vi "VolumeScan.vi"() -> ()   [LabVIEW 2018]
uses:
  <vilib>/Utility/miscctls.llb/LVRowAndColumnTypeDef.ctl
  <vilib>/vision/NI_Vision_Development_Module.lvlib
panel:
  in  "Graph parameters":T1={"Graph type"=1, "Scale"=1.0, "Offset"=0.0, "Automatic"=""} {"Graph type" items=["Mean(Y)", "Mean(X)"]}
  out "Image":T2(plugin-control)
  out "XY Graph":cluster{"X":dbl, "Y":dbl}[](graph)
  out "Status":string
  in  "Capture":bool
  in  "Tab Control":T3(tab)
  in  "Graph settings":bool
  in  "Close camera":bool
  in  "Display":u16(ring) items=["Image", "Graph", "Volume"]
  in  "Frames per position":u32=1 min=1 step=1
  in  "Camera settings":bool
  out "Status":bool
  out "Temperature":dbl
  in  "Camera identity":u16(ring)=1 items=["Andor", "Dummy", "PCO Edge", "PointGrey Grasshopper Temp", "PointGrey Grasshopper"]
  in  "Exposure (s)":dbl=0.1
  in  "16-bit mapping":u16(ring) items=["Full range", "Full dynamic", "90% dynamic", "Fixed"]
  in  "16 bit low":i32
  in  "16 bit high":i32=65535
  in  "Camera settings table":i32(listbox)=-1
  in  "Open camera":bool
  in  "Wizards":i32(ring) items=["Circle", "Function"]
  in  "Volume Wizard":bool
  in  "Imaging Locations":dbl[][](array[numeric])
  in  "Device positions":dbl[](array[numeric]) format="%_5g"
  in  "Save":T4(ring)
  in  "Path":path=path "G:/"
  in  "File Prefix":string="Prefix"
  in  "Configure device":bool
  in  "Close device":bool
  in  "Device Settings":i32(listbox)=-1
  in  "Open device":bool
  in  "Shut Down":bool
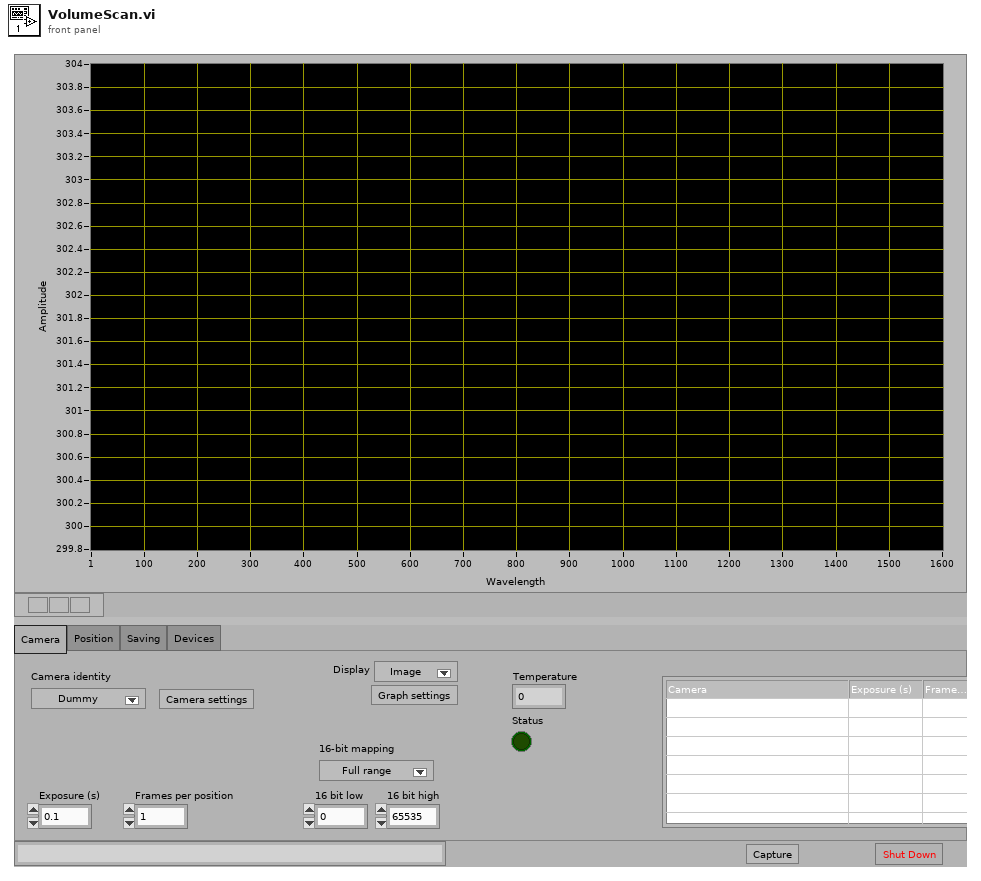
[diagram p1: front panel]
types:
  T1 = cluster{"Graph type":u16, "Scale":dbl, "Offset":dbl, "Automatic":string}
  T2 = typedef "IMAQ Image.ctl" = refnum<image>
  T3 = enum32{"Camera", "Position", "Saving", "Devices"}
  T4 = enum16{"Don't save", "Save U16", "Save PNG", "Save TIFF"}
  T5 = typedef "LVRowAndColumnTypeDef.ctl" = cluster{"Row":i32, "Column":i32}
  T6 = enum16{"Initialize", "Shut down", "Set capture mode", "Set exposure", "Trigger and read", "Get status", "Other settings"}
  T7 = typedef "Image Type" = u32
  T8 = enum16{"Initialize", "Shut down", "Set position", "Get position", "Get status", "Other settings"}
  T9 = cluster{"System OK?":bool, "Current exposure":dbl, "Temperature":dbl, "ROI":cluster{"X":u32, "X2":u32, "Y":u32, "Y2":u32}, "Binning":cluster{"X":u32, "Y":u32}}
  T10 = cluster{"System OK?":bool, "Temperature":dbl, "Limit switch high":bool[], "Limit switch low":bool[]}
  T11 = typedef "LVPoint32TypeDef.ctl" = cluster{"Horizontal":i32, "Vertical":i32}
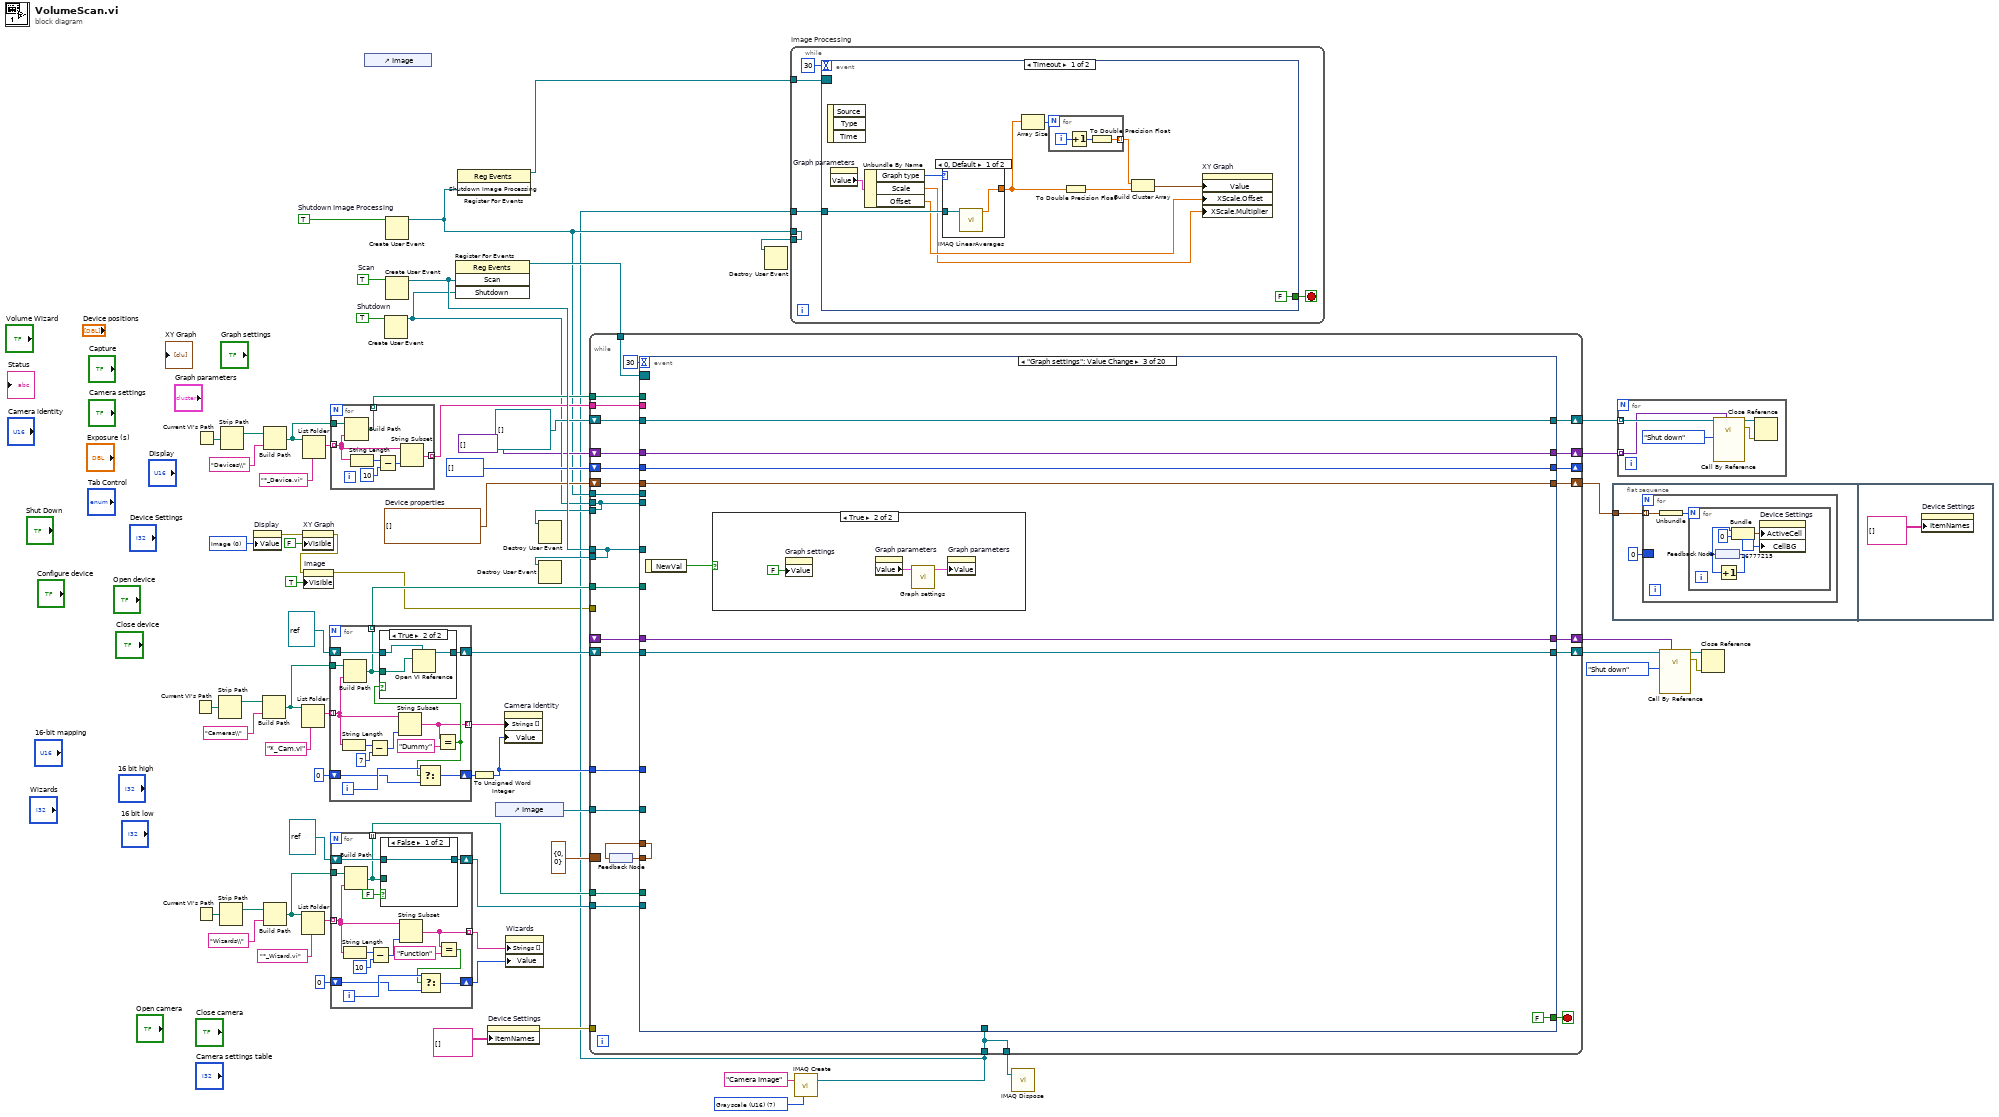
[diagram p0: block diagram]
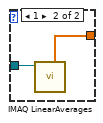
[diagram p2: hidden frame]
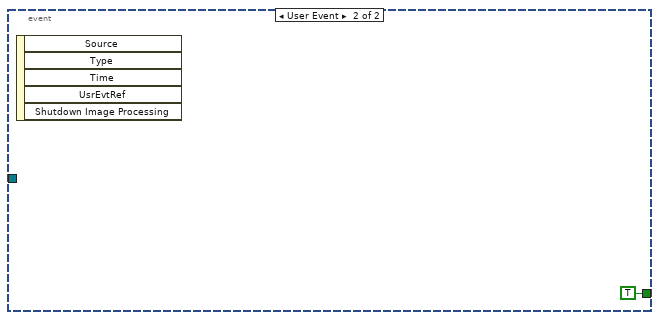
[diagram p3: hidden frame]
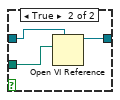
[diagram p4: hidden frame]
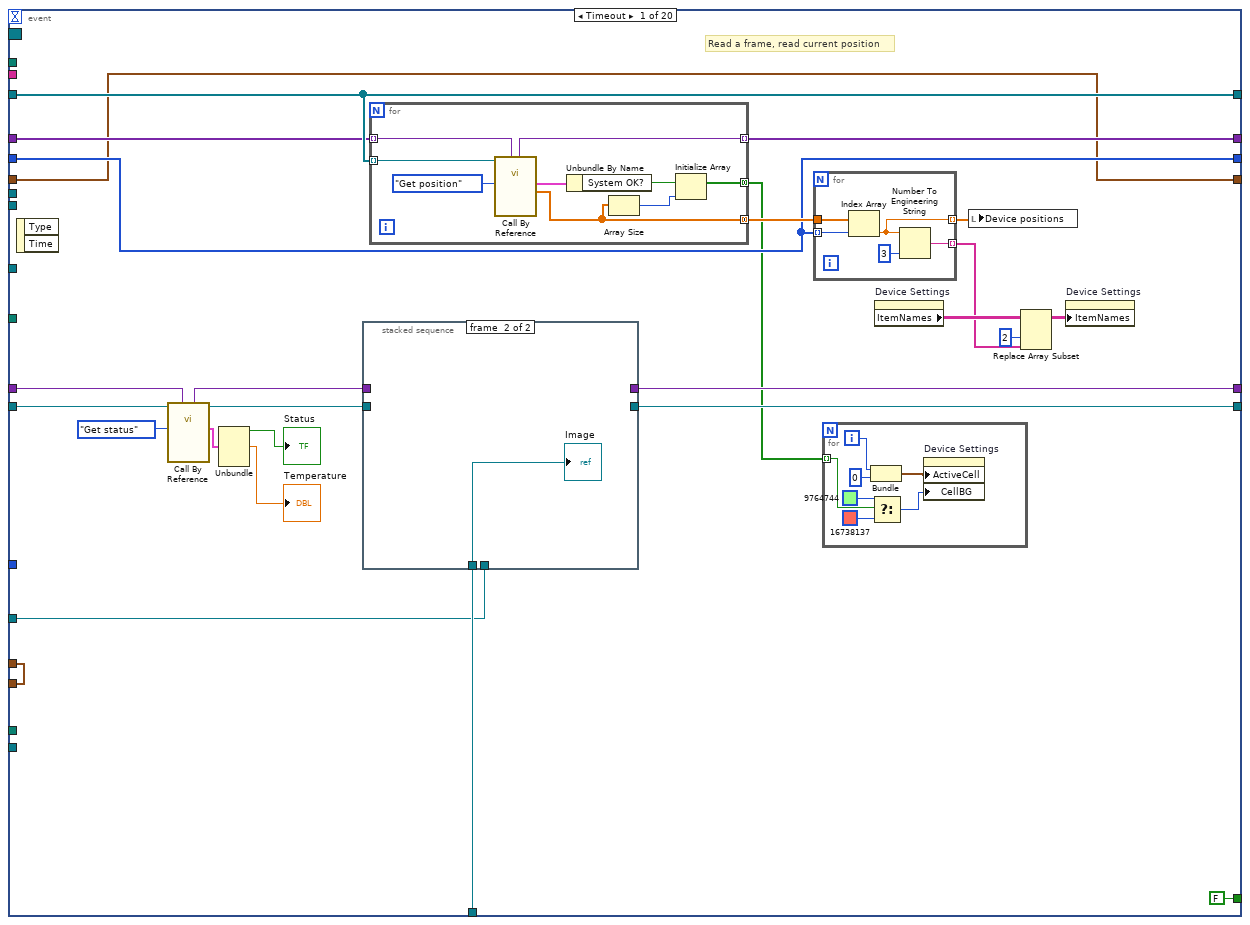
[diagram p6: hidden frame]
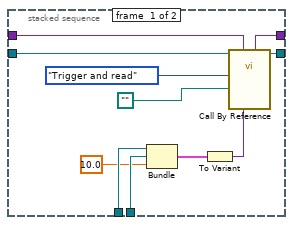
[diagram p7: hidden frame]
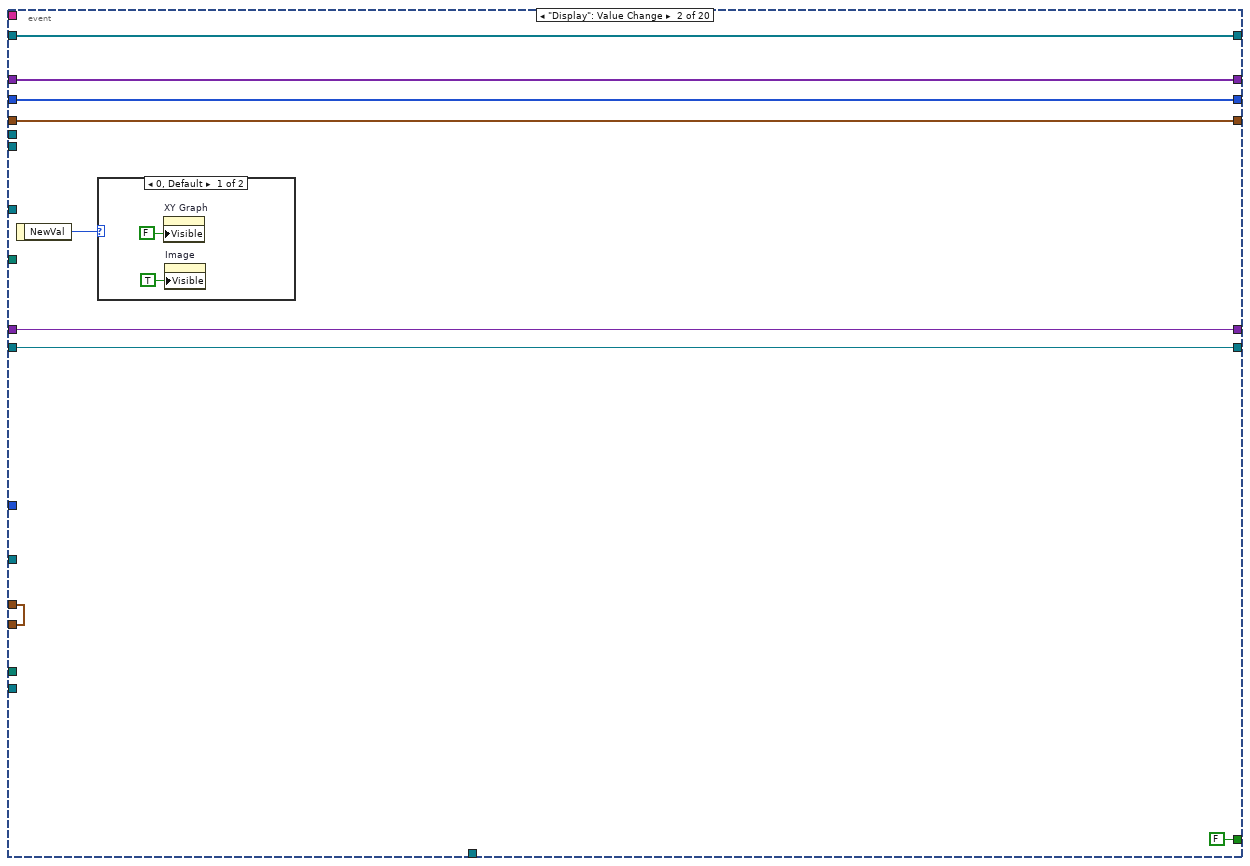
[diagram p8: hidden frame]
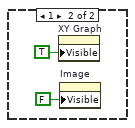
[diagram p9: hidden frame]
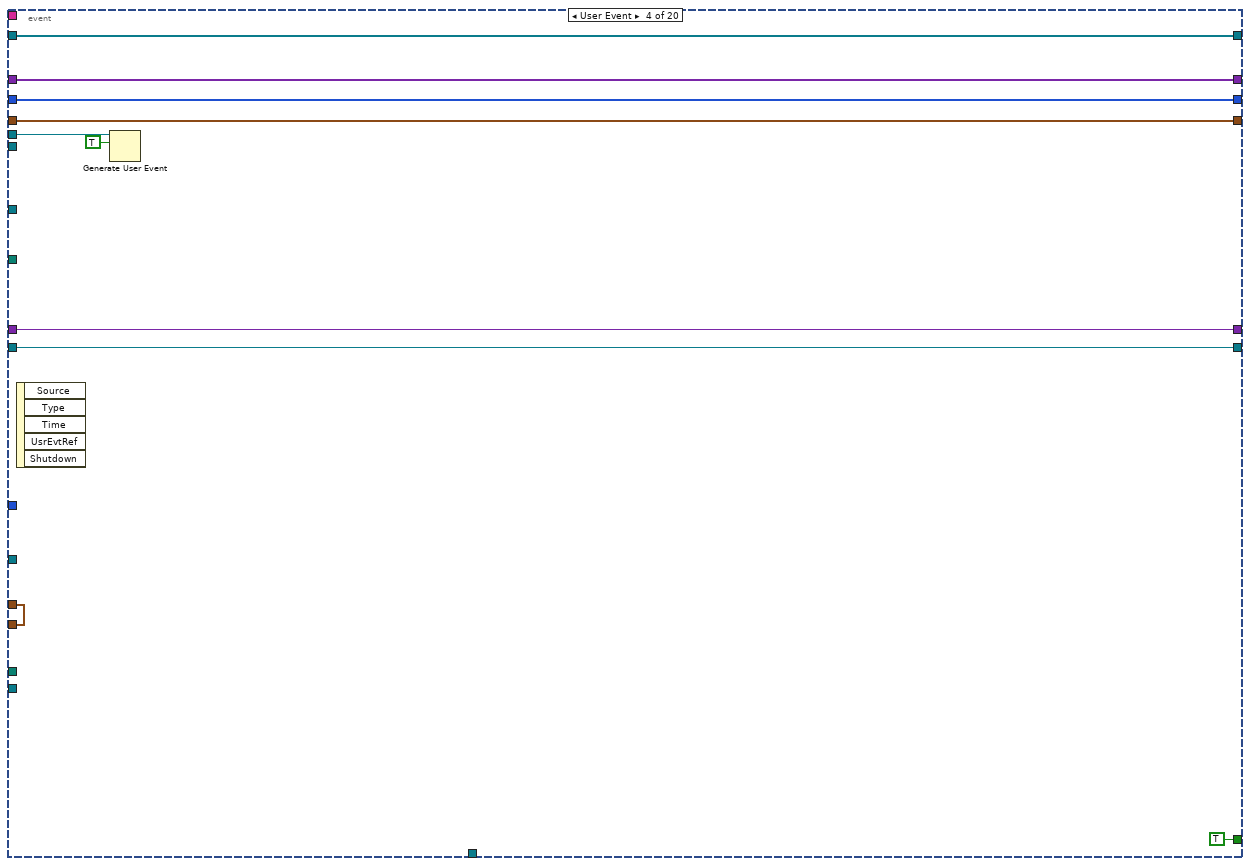
[diagram p11: hidden frame]
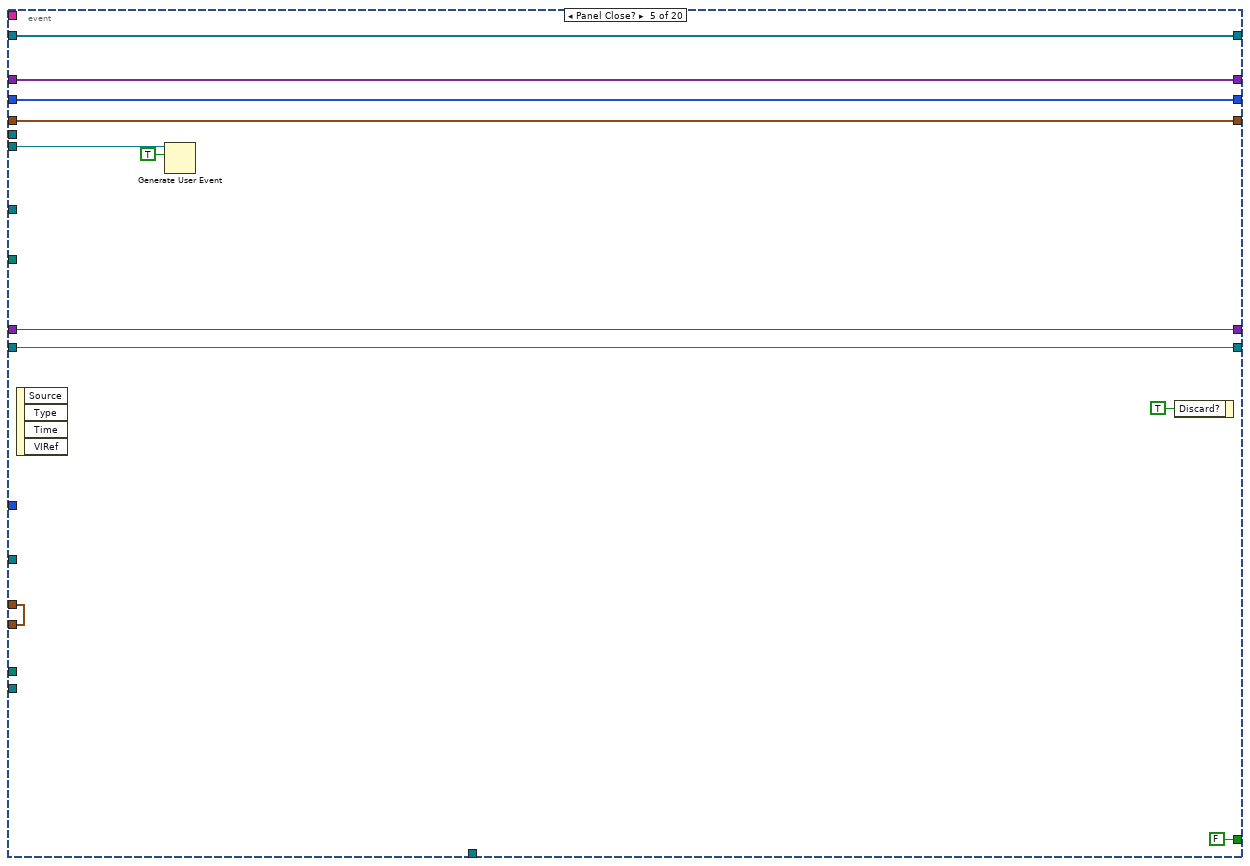
[diagram p12: hidden frame]
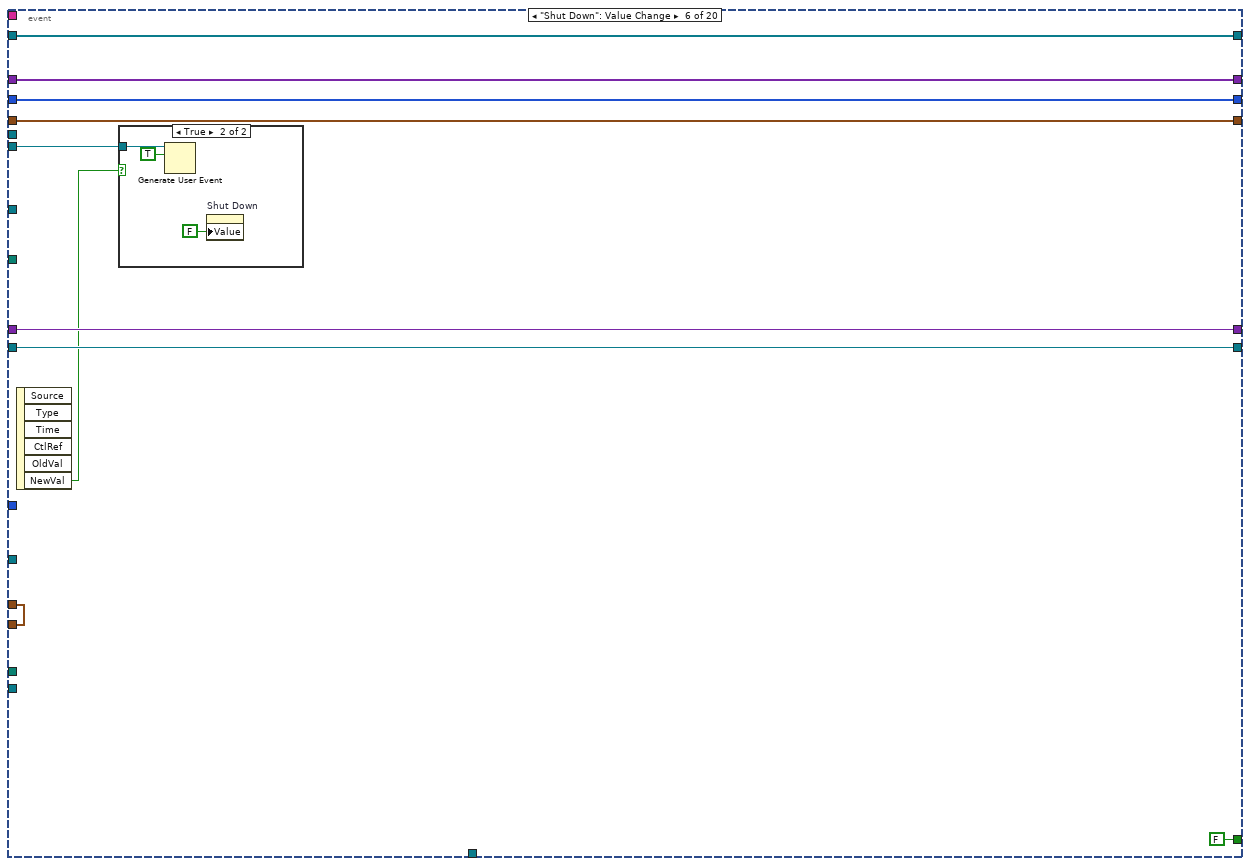
[diagram p13: hidden frame]
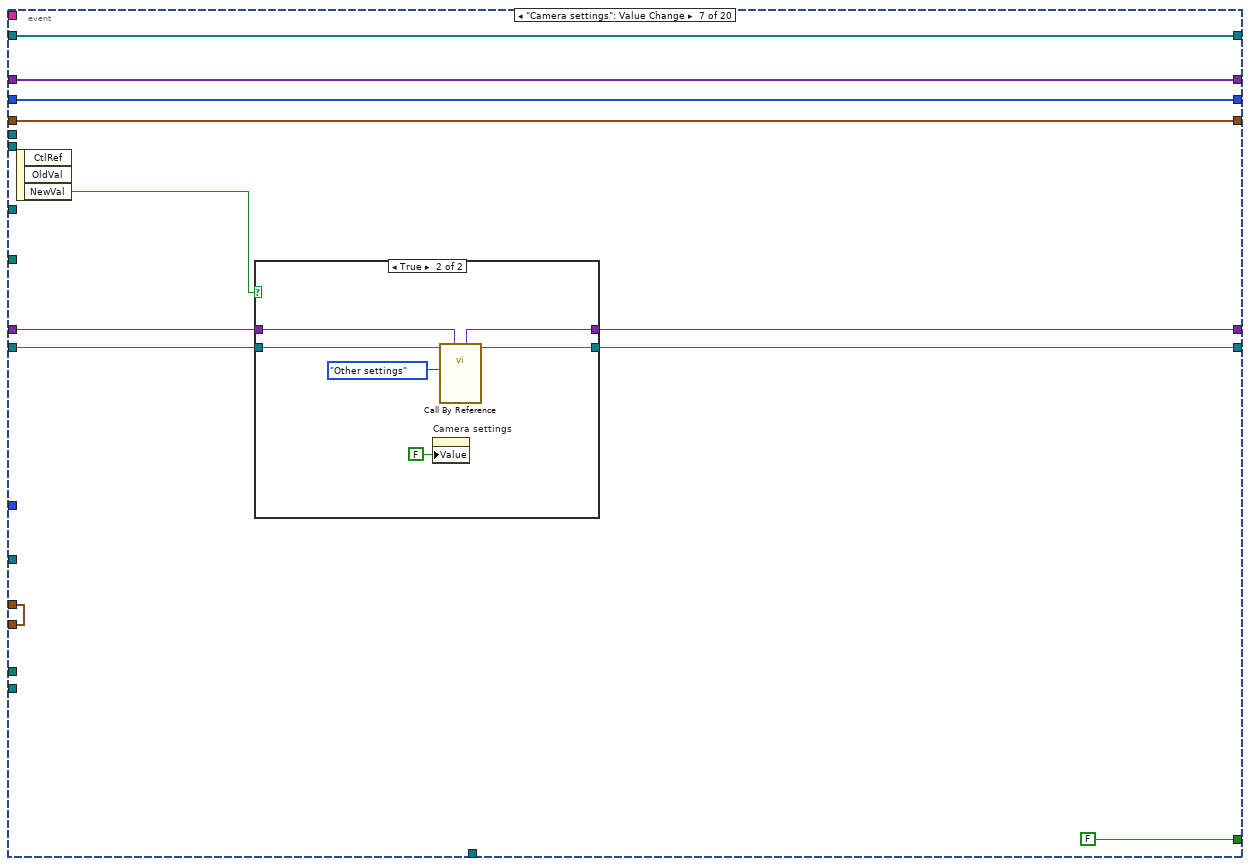
[diagram p15: hidden frame]
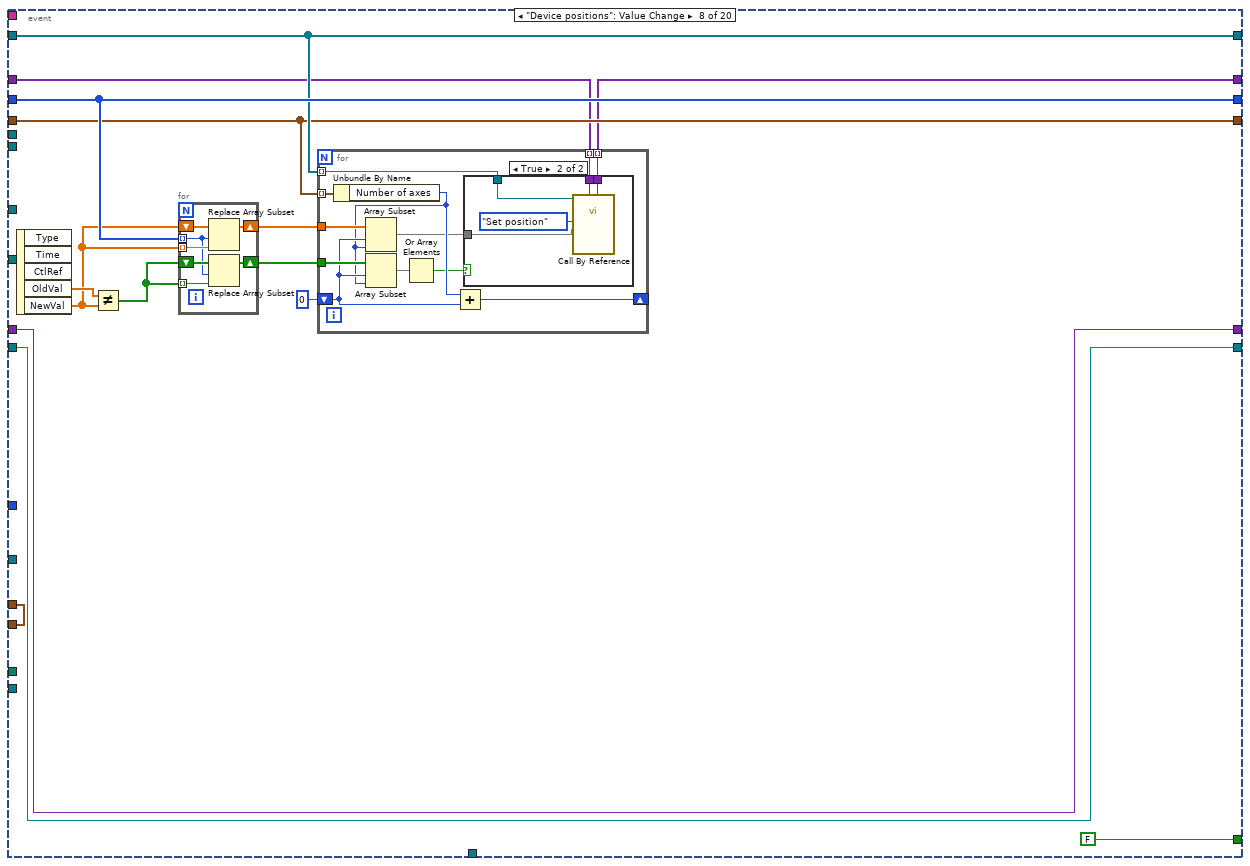
[diagram p17: hidden frame]
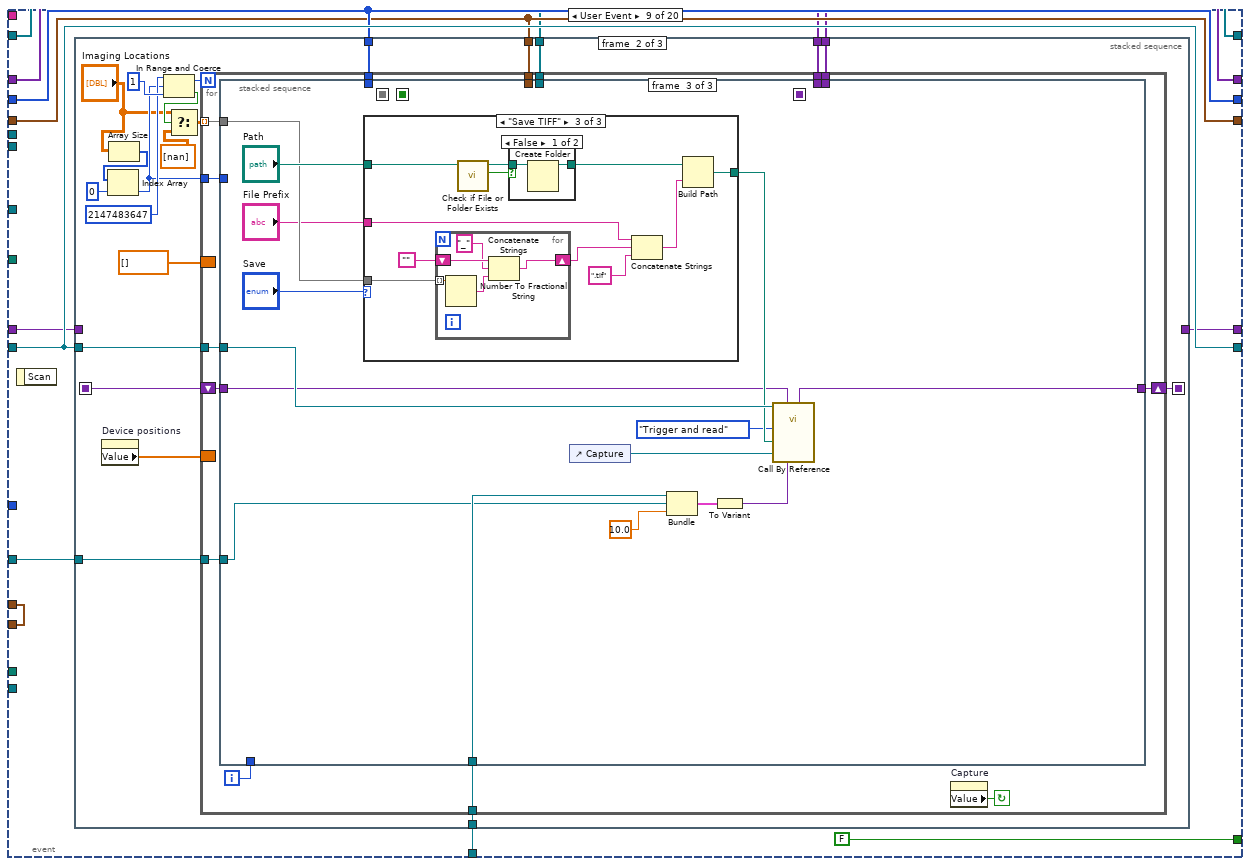
[diagram p19: hidden frame]
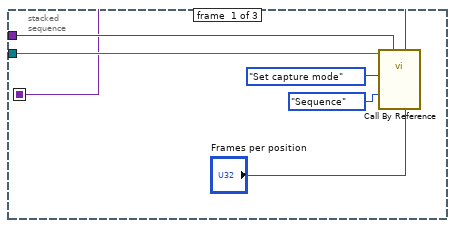
[diagram p20: hidden frame]
diagram:
  w6 = u16 0 items=["Image", "Graph", "Volume"] ("Display")
  w11 = TRUE  # Shutdown Image Processing
  w33 = TRUE  # Shutdown
  w36 = cluster{"Number of axes":i32}[] []  # Device properties
  w51 = T7 7 items=["Grayscale (U8)", "Grayscale (I16)", "Grayscale (SGL)", "Complex (CSG)", "RGB (U32)", "HSL (U32)", "RGB (U64)", "Grayscale (U16)"] ("Image Type")
  w70 = TRUE  # Scan
  n1 = Current VI's Path() -> (path=w67:path)
  n2 = Current VI's Path() -> (path=w16:path)
  n3 = Current VI's Path() -> (path=w41:path)
  n4 = Strip Path(path=w67) -> (stripped path=w66:path)  [unwired: 1 out]
  n5 = Strip Path(path=w16) -> (stripped path=w17:path)  [unwired: 1 out]
  n6 = Strip Path(path=w41) -> (stripped path=w42:path)  [unwired: 1 out]
  n7 = property on="Display" class="Ring (strict)"("Value"=w6) -> (error out=w3:errorcluster)  [unwired: 2 in, 1 out]
  n8 = Build Path(base path=w66, name or relative path="Cameras\\") -> (appended path=w59:path)
  n9 = Build Path(base path=w17, name or relative path="Wizards\\") -> (appended path=w22:path)
  n10 = Build Path(base path=w42, name or relative path="Devices\\") -> (appended path=w46:path)
  n11 = List Folder(path=w59, pattern="*_Cam.vi") -> (filenames=w63:string[])  [unwired: 2 in, 3 out]
  n12 = List Folder(path=w22, pattern="*_Wizard.vi") -> (filenames=w20:string[])  [unwired: 2 in, 3 out]
  n13 = List Folder(path=w46, pattern="*_Device.vi") -> (filenames=w45:string[])  [unwired: 2 in, 3 out]
  n14 = property on="XY Graph" class="XYGraph (strict)"(error in=w3, "Visible"=FALSE) -> (error out=w2:errorcluster)  [unwired: 1 in, 1 out]
  n15 = property on="Image" class="ImageControl"(error in=w2, "Visible"=TRUE) -> (error out=w1:errorcluster)  [unwired: 1 in, 1 out]
  n16 = for {
    tunnel: w63 -> [w71] mode=indexing
    tunnel: [w73] -> w62 mode=indexing
    shift-right: [w82] -> w60
    shift-left: 0 -> [w81]
    tunnel: w59 -> [w77]
    shift-right: [w79] -> w58
    shift-left: refnum<vi> refnum ("type specifier VI Refnum (for type only)") -> [w78]
    tunnel: [w76] -> w56 mode=indexing
    i -> [w83]
    n17 = String Length(string=w71) -> (length=w75:i32)
    n18 = Build Path(base path=w77, name or relative path=w71) -> (appended path=w76:path)
    n19 = Subtract(x=w75, y=7) -> (x-y=w72:i32)
    n20 = String Subset(string=w71, length (rest)=w72) -> (substring=w73:string)  [unwired: 1 in]
    n21 = Equal?(x=w73, y="Dummy") -> (x = y?=w80:bool)
    n22 = case shown="True" w80 {
      tunnel: [w85 w88] -> w79
      tunnel: w78 -> [w85 w86]
      tunnel: w76 -> [_ w87]
      frame False {
      }
      frame True {
        n23 = Open VI Reference(type specifier VI Refnum (for type only)=w86, vi path=w87) -> (vi reference=w88:refnum<vi>)  [unwired: 4 in, 1 out]
      }
    }
    n24 = Select(t=w83, s=w80, f=w81) -> (s? t:f=w82:i32)
  }
  n25 = for {
    tunnel: w20 -> [w90] mode=indexing
    tunnel: [w92] -> w14 mode=indexing
    shift-right: [w101] -> w15
    shift-left: 0 -> [w100]
    tunnel: w22 -> [w96]
    shift-right: [w98] -> w12
    shift-left: refnum<vi> refnum ("type specifier VI Refnum (for type only)") -> [w97]
    tunnel: [w95] -> w13 mode=indexing
    i -> [w102]
    n26 = String Length(string=w90) -> (length=w94:i32)
    n27 = Build Path(base path=w96, name or relative path=w90) -> (appended path=w95:path)
    n28 = Subtract(x=w94, y=10) -> (x-y=w91:i32)
    n29 = case shown="False" FALSE {
      tunnel: [w104 w107] -> w98
      tunnel: w97 -> [w104 w105]
      tunnel: w95 -> [_ w106]
      frame False {
      }
      frame True {
        n30 = Open VI Reference(type specifier VI Refnum (for type only)=w105, vi path=w106) -> (vi reference=w107:refnum<vi>)  [unwired: 4 in, 1 out]
      }
    }
    n31 = String Subset(string=w90, length (rest)=w91) -> (substring=w92:string)  [unwired: 1 in]
    n32 = Equal?(x=w92, y="Function") -> (x = y?=w99:bool)
    n33 = Select(t=w102, s=w99, f=w100) -> (s? t:f=w101:i32)
  }
  n34 = for {
    tunnel: w45 -> [w108] mode=indexing
    tunnel: [w110] -> w39 mode=indexing
    tunnel: w46 -> [w114]
    tunnel: [w113] -> w40 mode=indexing
    n35 = Build Path(base path=w114, name or relative path=w108) -> (appended path=w113:path)
    n36 = String Length(string=w108) -> (length=w112:i32)
    n37 = Subtract(x=w112, y=10) -> (x-y=w109:i32)
    n38 = String Subset(string=w108, length (rest)=w109) -> (substring=w110:string)  [unwired: 1 in]
  }
  n39 = control-ref of="Image"() -> ()  [unwired: 1 out]
  n40 = Create User Event(user event datatype=w33) -> (user event=w31:refnum<user-event>)  [unwired: 1 in, 1 out]
  n41 = Create User Event(user event datatype=w11) -> (user event=w8:refnum<user-event>)  [unwired: 1 in, 1 out]
  n42 = Create User Event(user event datatype=w70) -> (user event=w68:refnum<user-event>)  [unwired: 1 in, 1 out]
  n43 = register-events(w68, w31) -> (reference out=w69:refnum<event-registration>)  [unwired: 2 in, 1 out]
  n44 = register-events(w8) -> (reference out=w10:refnum<event-registration>)  [unwired: 2 in, 1 out]
  n45 = To Unsigned Word Integer(number=w60) -> (unsigned 16bit integer=w26:u16)
  n46 = property on="Device Settings" class="MCListbox (strict)"("ItemNames"=string[][] [] ("Device setup")) -> (error out=w28:errorcluster)  [unwired: 2 in, 1 out]
  n47 = control-ref of="Image"() -> (w47:refnum<vi>)
  n48 = property on="Camera identity" class="Ring (strict)"("Strings []"=w62, "Value"=w26) -> ()  [unwired: 2 in, 2 out]
  n49 = property on="Wizards" class="Ring (strict)"("Strings []"=w14, "Value"=w15) -> ()  [unwired: 2 in, 2 out]
  n50 = call "IMAQ Create"("Image Name"="Camera Image", "Image Type"=w51) -> ("New Image"=w7:T2)  [unwired: 3 in, 1 out]
  n51 = while {
    tunnel: w69 -> [w140]
    tunnel: w68 -> [w122]
    shift-right: [w139] -> w53
    shift-left: w58 -> [w138]
    tunnel: w56 -> [w137]
    tunnel: w7 -> [w136]
    tunnel: [w136] -> w50
    shift-right: [w135] -> w48
    shift-left: _ -> [w134]
    tunnel: w47 -> [w133]
    tunnel: w40 -> [w132]
    tunnel: w39 -> [w131]
    shift-right: [w130] -> w35
    shift-left: refnum<vi>[] [] ("appended array") -> [w129]
    shift-right: [w128] -> w34
    shift-left: variant[] [] -> [w127]
    shift-right: [w125] -> _
    shift-left: i32[] [] -> [w126]
    shift-right: [w124] -> w25
    shift-left: w36 -> [w123]
    tunnel: [w122] -> w32
    tunnel: w31 -> [w121]
    tunnel: [w121] -> w30
    tunnel: w28 -> [_]
    tunnel: w26 -> [w120]
    border: T5 {"Row"=0, "Column"=0} ("Cell Position") -> [_]
    tunnel: w13 -> [w117]
    tunnel: w12 -> [w116]
    tunnel: w8 -> [w115]
    tunnel: w1 -> [_]
    stop <- w141 stop-if-true
    n52 = feedback #1() -> (w118:T5)
    n53 = event shown="[2] \"Graph settings\": Value Change" {
      selector: w140 -> [_ _ _ _ _ _ _ _ _ _ _ _ _ _ _ _ _ _ _ _]
      dyn-events: _ -> [_ _ _ _ _ _ _ _ _ _ _ _ _ _ _ _ _ _ _ _]
      timeout: 30 -> [_ _ _ _ _ _ _ _ _ _ _ _ _ _ _ _ _ _ _ _]
      tunnel: [FALSE FALSE FALSE TRUE FALSE FALSE FALSE FALSE FALSE FALSE FALSE FALSE FALSE FALSE FALSE FALSE FALSE FALSE FALSE FALSE] -> w141
      tunnel: w122 -> [_ _ _ _ _ _ _ _ _ w582 _ _ _ _ _ _ _ _ _ _]
      tunnel: [w163 w204 w218 w234 w245 w255 w269 w292 w330 w580 w594 w628 w652 w667 w781 w889 w900 w925 w941 w1040] -> w139
      tunnel: w138 -> [w168 w204 w218 w234 w245 w255 w271 w292 w330 w580 w594 w635 w654 w667 w781 w889 w900 w925 w941 w1040]
      tunnel: w137 -> [_ _ _ _ _ _ _ _ _ _ _ w640 _ _ _ _ _ _ w931 _]
      tunnel: w136 -> [w158 _ _ _ _ _ _ _ w329 _ _ _ _ _ _ _ _ _ _ _]
      tunnel: [w159 w205 w219 w235 w246 w256 w267 w291 w327 w579 w593 w619 w647 w668 w782 w890 w901 w926 w942 w1041] -> w135
      tunnel: w134 -> [w161 w205 w219 w235 w246 w256 w266 w291 w328 w579 w593 w621 w648 w668 w782 w890 w901 w926 w942 w1041]
      tunnel: w133 -> [w157 _ _ _ _ _ _ _ w326 _ _ _ _ _ _ _ _ _ _ _]
      tunnel: w132 -> [_ _ _ _ _ _ _ _ _ _ _ _ _ w657 w771 _ _ _ _ _]
      tunnel: w131 -> [_ _ _ _ _ _ _ _ _ _ _ _ _ w666 w780 _ _ _ w940 _]
      tunnel: [w156 w209 w223 w230 w241 w251 w265 w287 w321 w578 w588 w618 w646 w658 w772 w881 w905 w928 w933 w1044] -> w130
      tunnel: w129 -> [w156 w209 w223 w230 w241 w251 w265 w287 w321 w578 w588 w618 w646 w662 w776 w881 w905 w928 w937 w1044]
      tunnel: [w155 w208 w222 w231 w242 w252 w263 w281 w322 w577 w589 w617 w645 w659 w773 w874 w904 w929 w934 w1045] -> w128
      tunnel: w127 -> [w154 w208 w222 w231 w242 w252 w263 w282 w323 w577 w589 w617 w645 w663 w777 w875 w904 w929 w930 w1045]
      tunnel: w126 -> [w151 w207 w221 w233 w244 w254 w264 w290 w325 w576 w592 w616 w644 w664 w778 w883 w903 w911 w938 w1043]
      tunnel: [w151 w207 w221 w233 w244 w254 w264 w290 w325 w576 w592 w616 w644 w660 w774 w883 w903 w910 w935 w1043] -> w125
      tunnel: [w150 w206 w220 w232 w243 w253 w262 w284 w324 w575 w590 w615 w643 w661 w775 w882 w902 w927 w936 w1042] -> w124
      tunnel: w123 -> [w150 w206 w220 w232 w243 w253 w262 w284 w324 w575 w590 w615 w643 w665 w779 w882 w902 w927 w939 w1042]
      tunnel: w121 -> [_ _ _ _ w239 w250 _ _ _ _ _ _ _ _ _ _ _ _ _ _]
      tunnel: w120 -> [_ _ _ _ _ _ _ _ _ _ _ w611 _ _ _ _ _ _ _ _]
      tunnel: [w143 w203 w217 w229 w237 w248 w261 w280 w320 w574 w591 w610 w642 w656 w770 w887 w897 w921 w932 w1038] -> w119
      tunnel: w118 -> [w143 w203 w217 w229 w237 w248 w261 w280 w320 w574 w591 w610 w642 w656 w770 w887 _ w921 w932 w1038]
      tunnel: w117 -> [_ _ _ _ _ _ _ _ _ _ w587 _ _ _ _ _ _ _ _ _]
      tunnel: w116 -> [_ _ _ _ _ _ _ _ _ _ w586 _ _ _ _ _ _ _ _ _]
      tunnel: w115 -> [_ _ _ w227 _ _ _ _ _ _ _ _ _ _ _ _ _ _ _ _]
      event Timeout {
        # "Read a frame, read current position"
        n54 = event-data() -> ()  [unwired: 1 in, 2 out]
        n55 = call-by-ref "?"(reference=w168, "Operation"=T6."Get status", "Camera-specific in"=w161) -> (reference out=w167:refnum<vi>, "Camera-specific out"=w160:variant, "Status"=w166:T9)  [unwired: 13 in, 1 out]
        n56 = Unbundle(w166) -> ("System OK?"=→"Status":bool, "Temperature"=→"Temperature":dbl)  [unwired: 3 out]
        n57 = stacked-sequence {
          tunnel: w167 -> [w200 _]
          tunnel: [w199 _] -> w163
          tunnel: w160 -> [w196 _]
          tunnel: [w195 _] -> w159
          tunnel: w158 -> [w194 w201]
          tunnel: w157 -> [w192 _]
          frame #0 {
            n58 = Bundle("New Image"=w194, "Image"=w192, 10.0) -> (w193:cluster{"New Image":T2, "Image":refnum<vi>, dbl})  [unwired: 1 in]
            n59 = To Variant(anything=w193) -> (Variant=w191:variant)
            n60 = call-by-ref "?"(reference=w200, "Operation"=T6."Trigger and read", "Camera-specific in"=w196, "Save path"=path "", "Image in"=w191) -> (reference out=w199:refnum<vi>, "Camera-specific out"=w195:variant)  [unwired: 11 in, 2 out]
          }
          frame #1 {
            "Image" <- w201
          }
        }
        n61 = for {
          tunnel: w156 -> [w189] mode=indexing
          tunnel: [w187] -> w155 mode=indexing
          tunnel: w154 -> [w186] mode=indexing
          tunnel: [w183] -> w144 mode=concatenating
          tunnel: [w182] -> w152 mode=concatenating
          n62 = call-by-ref "?"(reference=w189, "Device-specific in"=w186, "Operation"=T8."Get position") -> ("Position out"=w182:dbl[], "Status"=w185:T10, "Device-specific out"=w187:variant)  [unwired: 6 in, 4 out]
          n63 = Unbundle By Name(w185) -> ("System OK?"=w184:bool)
          n64 = Array Size(array=w182) -> (size(s)=w181:i32)
          n65 = Initialize Array(w184, w181) -> (w183:bool[])
        }
        n66 = for {
          tunnel: [w178] -> w153 mode=indexing
          tunnel: w152 -> [w180]
          tunnel: w151 -> [w179] mode=indexing
          tunnel: [w176] -> w146 mode=indexing
          n67 = Index Array(array=w180, index=w179) -> (element=w178:dbl)
          n68 = Number To Engineering String(2:i16 3 ("precision (6)"), 4:w178) -> (0:w176:string)  [unwired: 2 in]
        }
        n69 = for {
          tunnel: w144 -> [w172] mode=indexing
          i -> [w174]
          n70 = Bundle(w174, "Row"=0) -> (w173:cluster{i32, "Row":i32})  [unwired: 1 in]
          n71 = Select(t=u32 9764744, s=w172, f=u32 16738137) -> (s? t:f=w171:u32)
          n72 = property on="Device Settings" class="MCListbox (strict)"("ActiveCell"=w173, "CellBG"=w171) -> ()  [unwired: 2 in, 2 out]
        }
        n73 = property on="Device Settings" class="MCListbox (strict)"() -> ("ItemNames"=w148:string[][])  [unwired: 2 in, 2 out]
        n74 = local write "Device positions"(w153) -> ()
        n75 = Replace Array Subset(array=w148, new element=w146, index (col)=2 ("disabled index (col)")) -> (w147:string[][])  [unwired: 1 in]
        n76 = property on="Device Settings" class="MCListbox (strict)"("ItemNames"=w147) -> ()  [unwired: 2 in, 2 out]
      }
      event "Display": Value Change {
        n77 = event-data() -> ("NewVal"=w210:u16)  [unwired: 1 in]
        n78 = case shown="0, Default" w210 {
          frame 0, Default {
            n79 = property on="XY Graph" class="XYGraph (strict)"("Visible"=FALSE) -> ()  [unwired: 2 in, 2 out]
            n80 = property on="Image" class="ImageControl"("Visible"=TRUE) -> ()  [unwired: 2 in, 2 out]
          }
          frame 1 {
            n81 = property on="XY Graph" class="XYGraph (strict)"("Visible"=TRUE) -> ()  [unwired: 2 in, 2 out]
            n82 = property on="Image" class="ImageControl"("Visible"=FALSE) -> ()  [unwired: 2 in, 2 out]
          }
        }
      }
      event "Graph settings": Value Change {
        n83 = event-data() -> ("NewVal"=w215:bool)  [unwired: 1 in]
        n84 = case shown="True" w215 {
          frame False {
          }
          frame True {
            n85 = property on="Graph settings" class="Bool (strict)"("Value"=FALSE ("Graph settings")) -> ()  [unwired: 2 in, 2 out]
            n86 = property on="Graph parameters" class="Clust (strict)"() -> ("Value"=w226:T1)  [unwired: 2 in, 2 out]
            n87 = call "Graph settings.vi"("Settings in"=w226) -> ("Settings out"=w225:T1)  [unwired: 10 in]
            n88 = property on="Graph parameters" class="Clust (strict)"("Value"=w225) -> ()  [unwired: 2 in, 2 out]
          }
        }
      }
      event User Event {
        n89 = event-data() -> ()  [unwired: 1 in, 5 out]
        n90 = Generate User Event(user event=w227, event data cluster=TRUE ("event data")) -> ()  [unwired: 2 in, 2 out]
      }
      event Panel Close? {
        n91 = event-data() -> ()  [unwired: 1 in, 4 out]
        n92 = Generate User Event(user event=w239, event data cluster=TRUE ("event data")) -> ()  [unwired: 2 in, 2 out]
        n93 = event-data("Discard?"=TRUE) -> ()  [unwired: 1 in, 1 out]
      }
      event "Shut Down": Value Change {
        n94 = event-data() -> ("NewVal"=w249:bool)  [unwired: 1 in, 5 out]
        n95 = case shown="True" w249 {
          tunnel: w250 -> [_ w260]
          frame False {
          }
          frame True {
            n96 = Generate User Event(user event=w260, event data cluster=TRUE ("event data")) -> ()  [unwired: 2 in, 2 out]
            n97 = property on="Shut Down" class="Bool (strict)"("Value"=FALSE ("Shut Down")) -> ()  [unwired: 2 in, 2 out]
          }
        }
      }
      event "Camera settings": Value Change {
        n98 = event-data() -> ("NewVal"=w268:bool)  [unwired: 1 in, 2 out]
        n99 = case shown="True" w268 {
          tunnel: w271 -> [w273 w279]
          tunnel: [w273 w278] -> w269
          tunnel: [w272 w275] -> w267
          tunnel: w266 -> [w272 w274]
          frame False {
          }
          frame True {
            n100 = property on="Camera settings" class="Bool (strict)"("Value"=FALSE ("Camera settings")) -> ()  [unwired: 2 in, 2 out]
            n101 = call-by-ref "?"(reference=w279, "Operation"=T6."Other settings", "Camera-specific in"=w274) -> (reference out=w278:refnum<vi>, "Camera-specific out"=w275:variant)  [unwired: 13 in, 2 out]
          }
        }
      }
      event "Device positions": Value Change {
        n102 = event-data() -> ("OldVal"=w293:dbl[], "NewVal"=w289:dbl[])  [unwired: 1 in, 3 out]
        n103 = Not Equal?(x=w293, y=w289) -> (x != y?=w288:bool[])
        n104 = for {
          shift-right: [w318] -> w285
          shift-left: w289 -> [w319]
          tunnel: w290 -> [w313] mode=indexing
          tunnel: w289 -> [w317] mode=indexing
          tunnel: w288 -> [w315] mode=indexing
          shift-right: [w314] -> w286
          shift-left: w288 -> [w316]
          n105 = Replace Array Subset(array=w319, new element=w317, index=w313) -> (w318:dbl[])
          n106 = Replace Array Subset(array=w316, new element=w315, index=w313) -> (w314:bool[])
        }
        n107 = for {
          tunnel: w287 -> [w297] mode=indexing
          tunnel: w282 -> [w296] mode=indexing
          tunnel: w286 -> [w304]
          tunnel: w285 -> [w303]
          shift-right: [w305] -> _
          shift-left: 0 -> [w302]
          tunnel: w284 -> [w306] mode=indexing
          tunnel: [w295] -> w281 mode=indexing
          n108 = Unbundle By Name(w306) -> ("Number of axes"=w301:i32)
          n109 = Array Subset(array=w303, index=w302, length=w301) -> (w298:dbl[])
          n110 = Array Subset(array=w304, index=w302, length=w301) -> (w300:bool[])
          n111 = Or Array Elements(Boolean array=w300) -> (logical OR=w299:bool)
          n112 = Add(x=w301, y=w302) -> (x+y=w305:i32)
          n113 = case shown="True" w299 {
            tunnel: w298 -> [_ w308]
            tunnel: w297 -> [_ w312]
            tunnel: w296 -> [w307 w311]
            tunnel: [w307 w310] -> w295
            frame False {
            }
            frame True {
              n114 = call-by-ref "?"(reference=w312, "Device-specific in"=w311, "Position in"=w308, "Operation"=T8."Set position") -> ("Device-specific out"=w310:variant)  [unwired: 5 in, 6 out]
            }
          }
        }
      }
      event User Event {
        n115 = event-data() -> ()  [unwired: 1 in, 1 out]
        n116 = stacked-sequence {
          seq-local: [w333 _ _] -> [_ w357 _]
          seq-local: [_ w356 _] -> [_ _ w569]
          tunnel: w330 -> [w337 w359 w571]
          tunnel: w329 -> [_ w358 _]
          tunnel: w328 -> [w334 _ _]
          tunnel: [_ _ w568] -> w327
          tunnel: w326 -> [_ w355 _]
          tunnel: w325 -> [_ w354 _]
          tunnel: w324 -> [_ w353 _]
          tunnel: w323 -> [_ w352 _]
          tunnel: [_ w351 _] -> w322
          tunnel: w321 -> [_ w350 _]
          frame #0 {
            n117 = call-by-ref "?"(reference=w337, "Operation"=T6."Set capture mode", "Camera-specific in"=w334, "Capture mode"=enum16{"Single frame", "Sequence"}."Sequence", "Frames in sequence"="Frames per position") -> ("Camera-specific out"=w333:variant)  [unwired: 11 in, 3 out]
          }
          frame #1 {
            n118 = property on="Device positions" class="Arr (strict)"() -> ("Value"=w338:dbl[])  [unwired: 2 in, 2 out]
            n119 = Array Size(array="Imaging Locations") -> (size(s)=w348:i32[])
            n120 = Index Array(array=w348, index=0) -> (element=w343:i32)
            n121 = In Range and Coerce(upper limit=2147483647, x=w343, lower limit=1) -> (coerced(x)=w346:i32, In Range?=w341:bool)
            n122 = Select(t="Imaging Locations", s=w341, f=dbl[][] [[nan]] ("Imaging Locations")) -> (s? t:f=w342:dbl[][])
            n123 = for {
              N: w346 -> [_]
              tunnel: w342 -> [w373] mode=indexing
              tunnel: w359 -> [w371]
              tunnel: w358 -> [w370]
              shift-right: [w368] -> w356
              shift-left: w357 -> [w369]
              tunnel: w355 -> [w367]
              tunnel: w354 -> [w366]
              tunnel: w353 -> [w365]
              tunnel: w352 -> [w364]
              tunnel: [w363] -> w351
              tunnel: w350 -> [w362]
              border: dbl[] [] ("Imaging Locations") -> [_]
              tunnel: w343 -> [w360]
              border: w338 -> [_]
              i -> [w361]
              stop <- w372 continue-if-true
              n124 = stacked-sequence {
                seq-local: [w377 _ _] -> [_ w438 _]
                seq-local: [w376 _ _] -> [_ w436 _]
                seq-local: [w375 _ _] -> [_ w437 _]
                tunnel: w373 -> [w379 _ w524]
                tunnel: w371 -> [_ _ w521]
                tunnel: w370 -> [_ _ w516]
                tunnel: w369 -> [_ _ w518]
                tunnel: [_ _ w517] -> w368
                tunnel: w367 -> [_ _ w515]
                tunnel: w366 -> [w384 _ _]
                tunnel: w365 -> [w383 w441 _]
                tunnel: w364 -> [w382 _ _]
                tunnel: [_ w440 _] -> w363
                tunnel: w362 -> [w381 w439 _]
                tunnel: w361 -> [w380 _ _]
                tunnel: w360 -> [w374 w435 _]
                frame #0 {
                  n125 = Equal To 0?(x=w380) -> (x = 0?=w378:bool)
                  n126 = case shown="1, Default" w374 {
                    tunnel: w384 -> [_ w402]
                    tunnel: w383 -> [_ w388]
                    tunnel: w382 -> [w385 w401]
                    tunnel: w381 -> [_ w389]
                    tunnel: w379 -> [_ w397]
                    tunnel: w378 -> [_ w395]
                    tunnel: [w385 w392] -> w377
                    tunnel: [_ w391] -> w376
                    tunnel: [_ w390] -> w375
                    frame 0 {
                    }
                    frame 1, Default {
                      n127 = Array Size(array=w397) -> (size(s)=w400:i32)
                      n128 = feedback #2() -> (w398:dbl[])
                      n129 = Not Equal?(x=w398, y=w397) -> (x != y?=w393:bool[])
                      n130 = feedback-in #2(w397) -> ()
                      n131 = Initialize Array(TRUE, w400) -> (w394:bool[])
                      n132 = Select(t=w394, s=w395, f=w393) -> (s? t:f=w396:bool[])
                      n133 = feedback #3() -> (w386:dbl[])
                      n134 = for {
                        shift-right: [w430] -> w391
                        shift-left: w397 -> [w434]
                        tunnel: w402 -> [w428] mode=indexing
                        tunnel: w397 -> [w427] mode=indexing
                        tunnel: w396 -> [w432] mode=indexing
                        shift-right: [w431] -> w390
                        shift-left: w396 -> [w433]
                        tunnel: w386 -> [w429]
                        tunnel: [w430] -> w387
                        n135 = Not A Number/Path/Refnum?(number/path/refnum=w427) -> (NaN/Path/Refnum?=w422:bool)
                        n136 = Index Array(array=w429, index=w428) -> (element=w426:dbl)
                        n137 = Not(x=w422) -> (.not. x?=w423:bool)
                        n138 = Select(t=w426, s=w422, f=w427) -> (s? t:f=w425:dbl)
                        n139 = And(x=w432, y=w423) -> (x .and. y?=w424:bool)
                        n140 = Replace Array Subset(array=w434, new element=w425, index=w428) -> (w430:dbl[])
                        n141 = Replace Array Subset(array=w433, new element=w424, index=w428) -> (w431:bool[])
                      }
                      n142 = feedback-in #3(w387) -> ()
                      n143 = property on="Device positions" class="Arr (strict)"("Value"=w387) -> ()  [unwired: 2 in, 2 out]
                      n144 = for {
                        tunnel: w389 -> [w407] mode=indexing
                        tunnel: w401 -> [w406] mode=indexing
                        tunnel: w390 -> [w413]
                        tunnel: w391 -> [w412]
                        shift-right: [w414] -> _
                        shift-left: 0 -> [w411]
                        tunnel: w388 -> [w415] mode=indexing
                        tunnel: [w405] -> w392 mode=indexing
                        n145 = Unbundle By Name(w415) -> ("Number of axes"=w410:i32)
                        n146 = Array Subset(array=w412, index=w411, length=w410) -> (w404:dbl[])
                        n147 = Array Subset(array=w413, index=w411, length=w410) -> (w409:bool[])
                        n148 = Or Array Elements(Boolean array=w409) -> (logical OR=w408:bool)
                        n149 = Add(x=w410, y=w411) -> (x+y=w414:i32)
                        n150 = case shown="True" w408 {
                          tunnel: w404 -> [_ w417]
                          tunnel: w407 -> [_ w421]
                          tunnel: w406 -> [w416 w420]
                          tunnel: [w416 w419] -> w405
                          frame False {
                          }
                          frame True {
                            n151 = call-by-ref "?"(reference=w421, "Device-specific in"=w420, "Position in"=w417, "Operation"=T8."Set position") -> ("Device-specific out"=w419:variant)  [unwired: 5 in, 6 out]
                          }
                        }
                      }
                    }
                  }
                }
                frame #1 {
                  n152 = case shown="1, Default" w435 {
                    tunnel: w441 -> [_ w450]
                    tunnel: [w442 w449] -> w440
                    tunnel: w439 -> [_ w448]
                    tunnel: w438 -> [w442 w447]
                    tunnel: w437 -> [_ w446]
                    tunnel: w436 -> [_ w445]
                    frame 0 {
                    }
                    frame 1, Default {
                      w443 = u32 3000  # Timeout (ms)
                      n153 = Tick Count (ms)() -> (millisecond timer value=w444:u32)
                      n154 = while {
                        tunnel: w450 -> [w464]
                        tunnel: w448 -> [w462]
                        tunnel: w446 -> [w460]
                        tunnel: w445 -> [w459]
                        shift-right: [w463] -> w449
                        shift-left: w447 -> [w461]
                        tunnel: w444 -> [w455]
                        tunnel: w443 -> [w451]
                        stop <- w453 continue-if-true
                        n155 = for {
                          tunnel: w462 -> [w473] mode=indexing
                          tunnel: w461 -> [w472] mode=indexing
                          tunnel: w459 -> [w477]
                          shift-right: [w478] -> _
                          shift-left: 0 -> [w466]
                          tunnel: w464 -> [w479] mode=indexing
                          tunnel: [w471] -> w463 mode=indexing
                          shift-right: [w469] -> w458
                          shift-left: w460 -> [w468]
                          n156 = Unbundle By Name(w479) -> ("Number of axes"=w476:i32)
                          n157 = Array Subset(array=w477, index=w466, length=w476) -> (w474:dbl[])
                          n158 = Array Subset(array=w468, index=w466, length=w476) -> (w470:bool[])
                          n159 = Or Array Elements(Boolean array=w470) -> (logical OR=w475:bool)
                          n160 = Add(x=w476, y=w466) -> (x+y=w478:i32)
                          n161 = case shown="True" w475 {
                            tunnel: w474 -> [_ w483]
                            tunnel: w473 -> [_ w494]
                            tunnel: w472 -> [w481 w493]
                            tunnel: [w481 w486] -> w471
                            tunnel: [w480 w487] -> w467
                            tunnel: w470 -> [w480 _]
                            frame False {
                            }
                            frame True {
                              n162 = call-by-ref "?"(reference=w494, "Device-specific in"=w493, "Operation"=T8."Get position") -> (reference out=w482:refnum<vi>, "Device properties"=w490:cluster{"Axes":string[], "Tolerance":dbl[][]}, "Position out"=w491:dbl[], "Device-specific out"=w485:variant)  [unwired: 6 in, 3 out]
                              n163 = Unbundle By Name(w490) -> ("Tolerance"=w489:dbl[][])
                              n164 = Subtract(x=w491, y=w483) -> (x-y=w488:dbl[])
                              n165 = for {
                                tunnel: w489 -> [w510] mode=indexing
                                tunnel: w488 -> [w503] mode=indexing
                                tunnel: [w504] -> w487 mode=indexing
                                n166 = Index Array(array=w510, index #1=1 ("index"), index #2=0 ("index")) -> (element #1=w508:dbl, element #2=w507:dbl)
                                n167 = In Range and Coerce(upper limit=w508, x=w503, lower limit=w507) -> (In Range?=w509:bool)  [unwired: 1 out]
                                n168 = Not A Number/Path/Refnum?(number/path/refnum=w503) -> (NaN/Path/Refnum?=w502:bool)
                                n169 = Not(x=w509) -> (.not. x?=w501:bool)
                                n170 = Or(x=w502, y=w501) -> (x .or. y?=w504:bool)
                              }
                              n171 = Or Array Elements(Boolean array=w487) -> (logical OR=w484:bool)
                              n172 = case shown="True" w484 {
                                tunnel: [w495 w500] -> w486
                                tunnel: w485 -> [w495 w499]
                                tunnel: w483 -> [_ w497]
                                tunnel: w482 -> [_ w496]
                                frame False {
                                }
                                frame True {
                                n173 = call-by-ref "?"(reference=w496, "Device-specific in"=w499, "Position in"=w497, "Operation"=T8."Set position") -> ("Device-specific out"=w500:variant)  [unwired: 5 in, 6 out]
                                }
                              }
                            }
                          }
                          n174 = Replace Array Subset(array=w468, new element=w467, index=w466) -> (w469:bool[])
                        }
                        n175 = Tick Count (ms)() -> (millisecond timer value=w456:u32)
                        n176 = call "Elapsed time.vi"("Start time (ms)"=w455, "Current time (ms)"=w456) -> ("Elapsed time"=w454:u32)
                        n177 = Less?(x=w454, y=w451) -> (x < y?=w452:bool)
                        n178 = Or Array Elements(Boolean array=w458) -> (logical OR=w457:bool)
                        n179 = And(x=w457, y=w452) -> (x .and. y?=w453:bool)
                      }
                    }
                  }
                }
                frame #2 {
                  n180 = case shown="\"Save TIFF\"" "Save" {
                    tunnel: "Path" -> [_ w543 w558]
                    tunnel: w524 -> [_ w538 w551]
                    tunnel: "File Prefix" -> [_ w532 w554]
                    tunnel: [path "" w527 w553] -> w520
                    frame "Don't save", Default {
                    }
                    frame "Save U16" {
                      w531 = "_"
                      n181 = Index Array(array=w538, index #1=0 ("index"), index #2=1 ("index"), index #3=2 ("index")) -> (element #1=w530:dbl, element #2=w529:dbl, element #3=w528:dbl)
                      n182 = call <vilib>:"Check if File or Folder Exists.vi"("path"=w543) -> ("file or folder exists?"=w542:bool, "dup path"=w541:path)  [unwired: 8 in, 1 out]
                      n183 = case shown="False" w542 {
                        tunnel: w541 -> [w547 w548]
                        tunnel: [w546 w548] -> w540
                        frame False {
                          n184 = Create Folder(path (use dialog)=w547) -> (created path=w546:path)  [unwired: 2 in, 2 out]
                        }
                        frame True {
                        }
                      }
                      n185 = Number To Fractional String(number=w530) -> (F-format string=w545:string)  [unwired: 3 in]
                      n186 = Number To Fractional String(number=w529) -> (F-format string=w534:string)  [unwired: 3 in]
                      n187 = Number To Fractional String(number=w528) -> (F-format string=w533:string)  [unwired: 3 in]
                      n188 = Concatenate Strings(w532, w531, w545, w531, w534, w531, w533, ".U16") -> (w544:string)
                      n189 = Build Path(base path=w540, name or relative path=w544) -> (appended path=w527:path)
                    }
                    frame "Save TIFF" {
                      n190 = for {
                        shift-right: [w560] -> w550
                        shift-left: "" -> [w564]
                        tunnel: w551 -> [w563] mode=indexing
                        n191 = Number To Fractional String(number=w563) -> (F-format string=w562:string)  [unwired: 3 in]
                        n192 = Concatenate Strings(w564, "_", w562) -> (w560:string)
                      }
                      n193 = call <vilib>:"Check if File or Folder Exists.vi"("path"=w558) -> ("file or folder exists?"=w557:bool, "dup path"=w556:path)  [unwired: 8 in, 1 out]
                      n194 = case shown="False" w557 {
                        tunnel: w556 -> [w566 w567]
                        tunnel: [w565 w567] -> w555
                        frame False {
                          n195 = Create Folder(path (use dialog)=w566) -> (created path=w565:path)  [unwired: 2 in, 2 out]
                        }
                        frame True {
                        }
                      }
                      n196 = Concatenate Strings(w554, w550, ".tif") -> (w559:string)
                      n197 = Build Path(base path=w555, name or relative path=w559) -> (appended path=w553:path)
                    }
                  }
                  n198 = control-ref of="Capture"() -> (w511:refnum<vi>)
                  n199 = Bundle("New Image"=w516, "Image"=w515, 10.0) -> (w513:cluster{"New Image":T2, "Image":refnum<vi>, dbl})  [unwired: 1 in]
                  n200 = To Variant(anything=w513) -> (Variant=w512:variant)
                  n201 = call-by-ref "?"(reference=w521, "Operation"=T6."Trigger and read", "Camera-specific in"=w518, "Save path"=w520, "Capture button"=w511, "Image in"=w512) -> ("Camera-specific out"=w517:variant)  [unwired: 10 in, 3 out]
                }
              }
              n202 = property on="Capture" class="Bool (strict)"() -> ("Value"=w372:bool)  [unwired: 2 in, 2 out]
            }
          }
          frame #2 {
            n203 = call-by-ref "?"(reference=w571, "Operation"=T6."Set capture mode", "Camera-specific in"=w569, "Capture mode"=enum16{"Single frame", "Sequence"}."Single frame") -> ("Camera-specific out"=w568:variant)  [unwired: 12 in, 3 out]
            n204 = property on="Capture" class="Bool (strict)"("Value"=FALSE ("Capture")) -> ()  [unwired: 2 in, 2 out]
          }
        }
      }
      event "Capture": Value Change {
        n205 = event-data() -> ("NewVal"=w583:bool)  [unwired: 1 in, 1 out]
        n206 = case shown="True" w583 {
          tunnel: w582 -> [_ w585]
          frame False {
          }
          frame True {
            n207 = Generate User Event(user event=w585, event data cluster=TRUE ("event data")) -> ()  [unwired: 2 in, 2 out]
          }
        }
      }
      event "Volume Wizard": Value Change {
        n208 = event-data() -> ("NewVal"=w596:bool)  [unwired: 1 in, 1 out]
        n209 = case shown="True" w596 {
          tunnel: w592 -> [_ w600]
          tunnel: w590 -> [_ w599]
          tunnel: w589 -> [_ w598]
          tunnel: w588 -> [_ w602]
          tunnel: w587 -> [_ w607]
          tunnel: w586 -> [_ w608]
          frame False {
          }
          frame True {
            n210 = property on="Wizards" class="Ring (strict)"() -> ("Value"=w605:i32)  [unwired: 2 in, 2 out]
            n211 = property on="Device Settings" class="MCListbox (strict)"() -> ("ItemNames"=w601:string[][])  [unwired: 2 in, 2 out]
            n212 = property on="Imaging Locations" class="Arr (strict)"() -> ("Value"=w597:dbl[][])  [unwired: 2 in, 2 out]
            n213 = Index Array(array=w607, index=w605) -> (element=w606:path)
            n214 = Open VI Reference(type specifier VI Refnum (for type only)=w608, vi path=w606) -> (vi reference=w604:refnum<vi>)  [unwired: 4 in, 1 out]
            n215 = call-by-ref "?"(reference=w604, "Input"=w597, "Device References"=w602, "Device properties"=w599, "Device parameters"=w598, "Device order"=w600, "Device description"=w601) -> ("Output"=w603:dbl[][])  [unwired: 6 in, 2 out]
            n216 = property on="Imaging Locations" class="Arr (strict)"("Value"=w603) -> ()  [unwired: 2 in, 2 out]
            n217 = property on="Volume Wizard" class="Bool (strict)"("Value"=FALSE ("Volume Wizard")) -> ()  [unwired: 2 in, 2 out]
          }
        }
      }
      event "Camera identity": Value Change {
        n218 = event-data() -> ("NewVal"=w639:u16)  [unwired: 1 in, 2 out]
        n219 = call <vilib>:"Set Busy.vi"() -> ("error out"=w626:errorcluster)  [unwired: 10 in, 1 out]
        n220 = call-by-ref "?"(reference=w635, error in=w626, "Operation"=T6."Shut down", "Camera-specific in"=w621) -> (reference out=w634:refnum<vi>, error out=w633:errorcluster)  [unwired: 12 in, 2 out]
        n221 = Close Reference(reference=w634, error in (no error)=w633) -> ()  [unwired: 1 out]
        n222 = Index Array(array=w640, index=w639) -> (element=w638:path)
        n223 = Open VI Reference(type specifier VI Refnum (for type only)=w634, vi path=w638) -> (vi reference=w637:refnum<vi>, error out=w614:errorcluster)  [unwired: 4 in]
        n224 = property on="Exposure (s)" class="DigNum (strict)"() -> ("Value"=w631:dbl)  [unwired: 2 in, 2 out]
        n225 = call-by-ref "?"(reference=w637, error in=w614, "Operation"=T6."Initialize", "Exposure time (s)"=w631) -> (reference out=w632:refnum<vi>, error out=w613:errorcluster, "Camera-specific out"=w620:variant, "Status"=w630:T9)  [unwired: 12 in]
        n226 = Unbundle By Name(w630) -> ("Current exposure"=w629:dbl)
        n227 = property on="Exposure (s)" class="DigNum (strict)"("Value"=w629) -> ()  [unwired: 2 in, 2 out]
        n228 = call-by-ref "?"(reference=w632, error in=w613, "Operation"=T6."Set capture mode", "Camera-specific in"=w620, "Capture mode"=enum16{"Single frame", "Sequence"}."Single frame") -> (reference out=w628:refnum<vi>, error out=w625:errorcluster, "Camera-specific out"=w619:variant)  [unwired: 11 in, 1 out]
        n229 = call <vilib>:"Unset Busy.vi"("error in (no error)"=w625) -> ("error out"=w612:errorcluster)  [unwired: 10 in]
        n230 = case shown="No Error" w612 {
          tunnel: w611 -> [_ w641]
          frame No Error {
          }
          frame Error {
            n231 = property on="Camera identity" class="Ring (strict)"("Val(Sgnl)"=w641) -> ()  [unwired: 2 in, 2 out]
          }
        }
      }
      event "Exposure (s)": Value Change {
        n232 = event-data() -> ("NewVal"=w653:dbl)  [unwired: 1 in, 2 out]
        n233 = call-by-ref "?"(reference=w654, "Operation"=T6."Set exposure", "Camera-specific in"=w648, "Exposure time (s)"=w653) -> (reference out=w652:refnum<vi>, "Camera-specific out"=w647:variant, "Status"=w651:T9)  [unwired: 12 in, 1 out]
        n234 = Unbundle By Name(w651) -> ("Current exposure"=w650:dbl)
        n235 = property on="Exposure (s)" class="DigNum (strict)"("Value"=w650) -> ()  [unwired: 2 in, 2 out]
      }
      event "Open device": Value Change {
        n236 = event-data() -> ("NewVal"=w669:bool)  [unwired: 1 in]
        n237 = case shown="True" w669 {
          tunnel: w666 -> [_ w675]
          tunnel: w665 -> [w671 w684]
          tunnel: w664 -> [w672 w683]
          tunnel: w663 -> [w673 w682]
          tunnel: w662 -> [w674 w681]
          tunnel: [w671 w680] -> w661
          tunnel: [w672 w679] -> w660
          tunnel: [w673 w678] -> w659
          tunnel: [w674 w677] -> w658
          tunnel: w657 -> [_ w676]
          frame False {
          }
          frame True {
            n238 = call "Select Device.vi"("Devices"=w675) -> ("Cancelled?"=w686:bool, "Device out"=w685:i32)  [unwired: 9 in]
            n239 = property on="Open device" class="Bool (strict)"("Value"=FALSE ("Open device")) -> ()  [unwired: 2 in, 2 out]
            n240 = case shown="False" w686 {
              tunnel: w685 -> [w709 _]
              tunnel: w684 -> [w699 w766]
              tunnel: w683 -> [w702 w767]
              tunnel: w682 -> [w714 w768]
              tunnel: w681 -> [w705 w769]
              tunnel: [w698 w766] -> w680
              tunnel: [w701 w767] -> w679
              tunnel: [w713 w768] -> w678
              tunnel: [w704 w769] -> w677
              tunnel: w676 -> [w719 _]
              tunnel: w675 -> [w710 _]
              frame False {
                n241 = Index Array(array=w710, index=w709) -> (element=w708:string)
                n242 = Index Array(array=w719, index=w709) -> (element=w718:path)
                n243 = Open VI Reference(type specifier VI Refnum (for type only)=refnum<vi> refnum, vi path=w718) -> (vi reference=w716:refnum<vi>, error out=w712:errorcluster)  [unwired: 4 in]
                n244 = property on="Device Settings" class="MCListbox (strict)"() -> ("ItemNames"=w707:string[][])  [unwired: 2 in, 2 out]
                n245 = flat-sequence {
                  tunnel: w712 -> [w720]
                  tunnel: w716 -> [w721]
                  tunnel: [w721] -> w689
                  tunnel: [w720] -> w688
                  tunnel: [w727] -> w693
                  tunnel: [w724] -> w692
                  tunnel: [w723] -> w691
                  tunnel: [w722] -> w690
                  tunnel: w689 -> [w728]
                  tunnel: w688 -> [w725]
                  tunnel: [w729] -> w694
                  tunnel: [w730] -> w703
                  tunnel: [w731] -> w711
                  tunnel: [w732] -> w715
                  tunnel: w693 -> [w732]
                  tunnel: w692 -> [w731]
                  tunnel: w691 -> [w730]
                  tunnel: w690 -> [w729]
                  frame #0 {
                    n246 = call <vilib>:"Set Busy.vi"() -> ()  [unwired: 10 in, 2 out]
                  }
                  frame #1 {
                    n247 = call-by-ref "?"(reference=w728, "error in (no error)"=w725, "Operation"=T8."Initialize") -> (reference out=w723:refnum<vi>, "Device properties"=w724:cluster{"Axes":string[], "Tolerance":dbl[][]}, "Position out"=w722:dbl[], "Device-specific out"=w727:variant)  [unwired: 6 in, 3 out]
                  }
                  frame #2 {
                    n248 = call <vilib>:"Unset Busy.vi"() -> ()  [unwired: 11 in, 1 out]
                  }
                }
                n249 = Unbundle By Name(w711) -> ("Axes"=w700:string[])
                n250 = for {
                  shift-right: [w748] -> w706
                  shift-left: w707 -> [w743]
                  tunnel: w700 -> [w752] mode=indexing
                  tunnel: w708 -> [w742]
                  tunnel: w694 -> [w751] mode=indexing
                  shift-right: [w734] -> w701
                  shift-left: w702 -> [w735]
                  n251 = Equal?(x=w742, y=w743) -> (x = y?=w745:bool[][])
                  n252 = Or Array Elements(Boolean array=w745) -> (logical OR=w744:bool)
                  n253 = case shown="True" w744 {
                    tunnel: w743 -> [_ w756]
                    tunnel: w742 -> [w753 w755]
                    tunnel: [w753 w754] -> w741
                    frame False {
                    }
                    frame True {
                      n254 = while {
                        tunnel: w756 -> [w763]
                        tunnel: w755 -> [w758]
                        tunnel: [w762] -> w754
                        i -> [w765]
                        stop <- w760 continue-if-true
                        n255 = call <vilib>:"Space Constant.vi"() -> ("String"=w757:string)
                        n256 = Increment(x=w765) -> (x+1=w759:i32)
                        n257 = Number To Decimal String(number=w759) -> (decimal integer string=w764:string)  [unwired: 1 in]
                        n258 = Concatenate Strings(w758, w757, w764) -> (w762:string)
                        n259 = Equal?(x=w762, y=w763) -> (x = y?=w761:bool[][])
                        n260 = Or Array Elements(Boolean array=w761) -> (logical OR=w760:bool)
                      }
                    }
                  }
                  n261 = Number To Exponential String(number=w751, precision (6)=i16 3) -> (E-format string=w750:string)  [unwired: 2 in]
                  n262 = Build Array(w741, w752, w750) -> (w749:string[])
                  n263 = Array Size(array=w743) -> (size(s)=w747:i32[])
                  n264 = Build Array(w749) -> (w737:string[][])
                  n265 = Index Array(array=w747, index=0) -> (element=w733:i32)
                  n266 = Bundle By Name(cluster=T5 {"Row"=0, "Column"=0} ("Active Cell:Active Cell"), "Row"=w733, "Column"=0 ("Row")) -> (w738:T5)
                  n267 = Insert Into Array(array=w743, index (row)=w733, new element=w737) -> (w748:string[][])  [unwired: 1 in]
                  n268 = Insert Into Array(array=w735, index=w733, new element=w733) -> (w734:i32[])
                  n269 = property on="Device Settings" class="MCListbox (strict)"("ActiveCell"=w738) -> ()  [unwired: 2 in, 2 out]
                }
                n270 = Array Size(array=w700) -> (size(s)=w696:i32)
                n271 = Build Array (concatenate)(w714, w715) -> (w713:variant[])
                n272 = Bundle By Name(cluster=cluster{"Number of axes":i32} {"Number of axes"=0}, "Number of axes"=w696) -> (w695:cluster{"Number of axes":i32})
                n273 = Build Array (concatenate)(w705, w703) -> (w704:refnum<vi>[])
                n274 = Build Array (concatenate)(w699, w695) -> (w698:cluster{"Number of axes":i32}[])
                n275 = property on="Device Settings" class="MCListbox (strict)"("ItemNames"=w706) -> ()  [unwired: 2 in, 2 out]
              }
              frame True {
              }
            }
          }
        }
      }
      event "Close device": Value Change {
        n276 = event-data() -> ("NewVal"=w783:bool)  [unwired: 1 in]
        n277 = case shown="True" w783 {
          tunnel: w780 -> [_ _]
          tunnel: w779 -> [w785 w793]
          tunnel: w778 -> [w786 w795]
          tunnel: w777 -> [w787 w797]
          tunnel: w776 -> [w788 w799]
          tunnel: [w785 w794] -> w775
          tunnel: [w786 w796] -> w774
          tunnel: [w787 w798] -> w773
          tunnel: [w788 w800] -> w772
          tunnel: w771 -> [_ _]
          frame False {
          }
          frame True {
            n278 = property on="Device Settings" class="MCListbox (strict)"() -> ("Value"=w789:i32, "ItemNames"=w792:string[][])  [unwired: 2 in, 2 out]
            n279 = property on="Close device" class="Bool (strict)"("Value"=FALSE ("Open device")) -> ()  [unwired: 2 in, 2 out]
            n280 = Greater Or Equal To 0?(x=w789) -> (x >= 0?=w790:bool)
            n281 = case shown="True" w790 {
              tunnel: w792 -> [_ w811]
              tunnel: [FALSE ("T button?") w806] -> w791
              tunnel: w789 -> [_ w805]
              frame False {
                n282 = One Button Dialog(message="Please select a valid device") -> ()  [unwired: 1 in, 1 out]
              }
              frame True {
                n283 = Index Array(array=w811, index (row)=w805, index (col)=0 ("disabled index (col)")) -> (element=w808:string)
                n284 = Concatenate Strings("Close device ", w808, "?" ("string")) -> (w804:string)
                n285 = Two Button Dialog(message=w804) -> (T button?=w806:bool)  [unwired: 2 in]
              }
            }
            n286 = case shown="True" w791 {
              tunnel: [w815 w836] -> w800
              tunnel: w799 -> [w815 w837]
              tunnel: [w814 w832] -> w798
              tunnel: w797 -> [w814 w833]
              tunnel: [w813 w824] -> w796
              tunnel: w795 -> [w813 w826]
              tunnel: [w812 w830] -> w794
              tunnel: w793 -> [w812 w831]
              tunnel: w789 -> [_ w839]
              frame False {
              }
              frame True {
                w816 = 0 ("index")
                w835 = 1 ("length")
                n287 = Index Array(array=w826, index=w839) -> (element=w838:i32)
                n288 = for {
                  shift-right: [w870] -> _
                  shift-left: w838 -> [w869]
                  tunnel: w831 -> [w872] mode=indexing
                  tunnel: [w873] -> w834
                  tunnel: [w868] -> w828 mode=indexing
                  tunnel: [w868] -> w829
                  i -> [w873]
                  stop <- w871 stop-if-true
                  n289 = Unbundle(w872) -> ("Number of axes"=w868:i32)
                  n290 = Subtract(x=w869, y=w868) -> (x-y=w870:i32)
                  n291 = Less Than 0?(x=w870) -> (x < 0?=w871:bool)
                }
                n292 = Add Array Elements(numeric array=w828) -> (sum=w827:i32)
                n293 = Decrement(x=w827) -> (x-1=w825:i32)
                n294 = for {
                  N: w829 -> [_]
                  tunnel: w825 -> [w848]
                  shift-right: [w846] -> w824
                  shift-left: w826 -> [w845]
                  i -> [w849]
                  n295 = Subtract(x=w848, y=w849) -> (x-y=w847:i32)
                  n296 = for {
                    tunnel: w847 -> [w851]
                    shift-right: [w854] -> w846
                    shift-left: i32[] [] -> [w855]
                    tunnel: w845 -> [w852] mode=indexing
                    tunnel: [w850] -> w843
                    i -> [w850]
                    n297 = Equal?(x=w851, y=w852) -> (x = y?=w853:bool)
                    n298 = case shown="False" w853 {
                      tunnel: w855 -> [w862 w867]
                      tunnel: [w861 w867] -> w854
                      tunnel: w852 -> [w857 _]
                      tunnel: w851 -> [w856 _]
                      tunnel: w850 -> [_ w863]
                      frame False {
                        n299 = Less?(x=w857, y=w856) -> (x < y?=w858:bool)
                        n300 = Decrement(x=w857) -> (x-1=w859:i32)
                        n301 = Select(t=w857, s=w858, f=w859) -> (s? t:f=w860:i32)
                        n302 = Build Array (concatenate)(w862, w860) -> (w861:i32[])
                      }
                      frame True {
                        n303 = property on="Device Settings" class="MCListbox (strict)"() -> ("ItemNames"=w866:string[][])  [unwired: 2 in, 2 out]
                        n304 = Delete From Array(array=w866, length=1, index (row)=w863) -> (array with subset deleted=w865:string[][])  [unwired: 1 in, 1 out]
                        n305 = property on="Device Settings" class="MCListbox (strict)"("ItemNames"=w865) -> ()  [unwired: 2 in, 2 out]
                      }
                    }
                  }
                  n306 = Bundle(w843, 0) -> (w841:cluster{i32, i32})  [unwired: 1 in]
                  n307 = property on="Device Settings" class="MCListbox (strict)"("ActiveCell"=w841, "CellBG"=u32 16777215) -> ()  [unwired: 2 in, 2 out]
                }
                n308 = Delete From Array(array=w837, length=w835, index=w834) -> (deleted portion=w819:refnum<vi>[], array with subset deleted=w836:refnum<vi>[])
                n309 = Delete From Array(array=w833, length=w835, index=w834) -> (deleted portion=w820:variant[], array with subset deleted=w832:variant[])
                n310 = Delete From Array(array=w831, length=w835, index=w834) -> (array with subset deleted=w830:cluster{"Number of axes":i32}[])  [unwired: 1 out]
                n311 = Index Array(array=w819, index=w816) -> (element=w818:refnum<vi>)
                n312 = Index Array(array=w820, index=w816) -> (element=w817:variant)
                n313 = call-by-ref "?"(reference=w818, "Device-specific in"=w817, "Operation"=T8."Shut down") -> (reference out=w822:refnum<vi>, error out=w823:errorcluster)  [unwired: 6 in, 5 out]
                n314 = Close Reference(reference=w822, error in (no error)=w823) -> ()  [unwired: 1 out]
              }
            }
          }
        }
      }
      event "Configure device": Value Change {
        n315 = event-data() -> ()  [unwired: 1 in, 6 out]
        n316 = property on="Configure device" class="Bool (strict)"("Value"=FALSE ("Configure device")) -> ()  [unwired: 2 in, 2 out]
        n317 = property on="Device Settings" class="MCListbox (strict)"() -> ("Value"=w884:i32)  [unwired: 2 in, 2 out]
        n318 = Index Array(array=w883, index=w884) -> (element=w885:i32)
        n319 = for {
          shift-right: [w893] -> _
          shift-left: w885 -> [w892]
          tunnel: w882 -> [w895] mode=indexing
          tunnel: [w896] -> w876
          i -> [w896]
          stop <- w894 stop-if-true
          n320 = Unbundle(w895) -> ("Number of axes"=w891:i32)
          n321 = Subtract(x=w892, y=w891) -> (x-y=w893:i32)
          n322 = Less Than 0?(x=w893) -> (x < 0?=w894:bool)
        }
        n323 = Index Array(array=w881, index=w876) -> (element=w878:refnum<vi>)
        n324 = Index Array(array=w875, index=w876) -> (element=w879:variant)
        n325 = call-by-ref "?"(reference=w878, "Device-specific in"=w879, "Operation"=T8."Other settings") -> ("Device-specific out"=w877:variant)  [unwired: 6 in, 6 out]
        n326 = Replace Array Subset(array=w875, new element=w877, index=w876) -> (w874:variant[])
      }
      event "Device Settings": Drag Starting {
        n327 = event-data() -> ("Coords"=w898:T11)  [unwired: 1 in, 4 out]
        n328 = invoke on="Device Settings" class="MCListbox (strict)" method="Point To Row Column"("Point"=w898) -> ("CellPosition"=w897:T5)  [unwired: 6 in, 6 out]
      }
      event "Device Settings": Drop {
        n329 = event-data() -> ("Coords"=w923:T11)  [unwired: 1 in, 5 out]
        n330 = invoke on="Device Settings" class="MCListbox (strict)" method="Point To Row Column"("Point"=w923) -> ("CellPosition"=w922:T5)  [unwired: 6 in, 6 out]
        n331 = Unbundle(w921) -> ("Row"=w913:i32)  [unwired: 1 out]
        n332 = Unbundle(w922) -> ("Row"=w909:i32)  [unwired: 1 out]
        n333 = In Range and Coerce(upper limit=2147483647, x=w909, lower limit=0) -> (coerced(x)=w908:i32)  [unwired: 1 out]
        n334 = property on="Device Settings" class="MCListbox (strict)"() -> ("ItemNames"=w920:string[][])  [unwired: 2 in, 2 out]
        n335 = Delete From Array(array=w920, length=1, index (row)=w913) -> (deleted portion=w917:string[][], array with subset deleted=w918:string[][])  [unwired: 1 in]
        n336 = Delete From Array(array=w911, length=1, index=w913) -> (deleted portion=w914:i32[], array with subset deleted=w915:i32[])
        n337 = Insert Into Array(array=w918, index (row)=w908, new element=w917) -> (w916:string[][])  [unwired: 1 in]
        n338 = Insert Into Array(array=w915, index=w908, new element=w914) -> (w910:i32[])
        n339 = property on="Device Settings" class="MCListbox (strict)"("ItemNames"=w916) -> ()  [unwired: 2 in, 2 out]
        n340 = event-data() -> ()  [unwired: 2 in, 1 out]
      }
      event "Open camera": Value Change {
        n341 = event-data() -> ("NewVal"=w943:bool)  [unwired: 1 in]
        n342 = disable-structure shown="Disabled" {
          disable-tunnel: w943 -> [w954 _]
          disable-tunnel: w940 -> [w953 _]
          disable-tunnel: w939 -> [w952 w1033]
          disable-tunnel: w938 -> [w951 w1034]
          disable-tunnel: w937 -> [w950 w1036]
          disable-tunnel: [w949 w1033] -> w936
          disable-tunnel: [w948 w1034] -> w935
          disable-tunnel: [w947 w1035] -> w934
          disable-tunnel: [w946 w1036] -> w933
          disable-tunnel: w931 -> [w945 _]
          disable-tunnel: w930 -> [_ w1035]
          frame Disabled {
            # "Currently work in progress - DO NOT USE"
            n343 = case shown="True" w954 {
              tunnel: w953 -> [_ w959]
              tunnel: w952 -> [w955 w968]
              tunnel: w951 -> [w956 w967]
              tunnel: _ -> [w957 w966]
              tunnel: w950 -> [w958 w965]
              tunnel: [w955 w964] -> w949
              tunnel: [w956 w963] -> w948
              tunnel: [w957 w962] -> w947
              tunnel: [w958 w961] -> w946
              tunnel: w945 -> [_ w960]
              frame False {
              }
              frame True {
                n344 = call "Select Device.vi"("Devices"=w959) -> ("Cancelled?"=w970:bool, "Device out"=w969:i32)  [unwired: 9 in]
                n345 = property on="Open camera" class="Bool (strict)"("Value"=FALSE ("Open device")) -> ()  [unwired: 2 in, 2 out]
                n346 = case shown="False" w970 {
                  tunnel: w969 -> [w990 _]
                  tunnel: w968 -> [w981 w1029]
                  tunnel: w967 -> [w983 w1030]
                  tunnel: w966 -> [w993 w1031]
                  tunnel: w965 -> [w986 w1032]
                  tunnel: [w980 w1029] -> w964
                  tunnel: [w982 w1030] -> w963
                  tunnel: [w992 w1031] -> w962
                  tunnel: [w985 w1032] -> w961
                  tunnel: w960 -> [w995 _]
                  tunnel: w959 -> [w991 _]
                  frame False {
                    w972 = dbl[] [] ("Position out")
                    n347 = property on="Camera settings table" class="MCListbox (strict)"() -> ("ItemNames"=w988:string[][])  [unwired: 2 in, 2 out]
                    n348 = Index Array(array=w991, index=w990) -> (element=w989:string)
                    n349 = Index Array(array=w995, index=w990) -> (element=w994:path)
                    n350 = Open VI Reference(type specifier VI Refnum (for type only)=refnum<vi> refnum, vi path=w994) -> (vi reference=w975:refnum<vi>)  [unwired: 4 in, 1 out]
                    n351 = for {
                      shift-right: [w1011] -> w987
                      shift-left: w988 -> [w1006]
                      tunnel: w972 -> [w1015] mode=indexing
                      tunnel: w989 -> [w1005]
                      tunnel: w972 -> [w1014] mode=indexing
                      shift-right: [w997] -> w982
                      shift-left: w983 -> [w998]
                      n352 = Equal?(x=w1005, y=w1006) -> (x = y?=w1008:bool[][])
                      n353 = Or Array Elements(Boolean array=w1008) -> (logical OR=w1007:bool)
                      n354 = case shown="True" w1007 {
                        tunnel: w1006 -> [_ w1019]
                        tunnel: w1005 -> [w1016 w1018]
                        tunnel: [w1016 w1017] -> w1004
                        frame False {
                        }
                        frame True {
                          n355 = while {
                            tunnel: w1019 -> [w1026]
                            tunnel: w1018 -> [w1021]
                            tunnel: [w1025] -> w1017
                            i -> [w1028]
                            stop <- w1023 continue-if-true
                            n356 = call <vilib>:"Space Constant.vi"() -> ("String"=w1020:string)
                            n357 = Increment(x=w1028) -> (x+1=w1022:i32)
                            n358 = Number To Decimal String(number=w1022) -> (decimal integer string=w1027:string)  [unwired: 1 in]
                            n359 = Concatenate Strings(w1021, w1020, w1027) -> (w1025:string)
                            n360 = Equal?(x=w1025, y=w1026) -> (x = y?=w1024:bool[][])
                            n361 = Or Array Elements(Boolean array=w1024) -> (logical OR=w1023:bool)
                          }
                        }
                      }
                      n362 = Number To Exponential String(number=w1014, precision (6)=i16 3) -> (E-format string=w1013:string)  [unwired: 2 in]
                      n363 = Build Array(w1004, w1015, w1013) -> (w1012:string[])
                      n364 = Array Size(array=w1006) -> (size(s)=w1010:i32[])
                      n365 = Build Array(w1012) -> (w1000:string[][])
                      n366 = Index Array(array=w1010, index=0) -> (element=w996:i32)
                      n367 = Bundle By Name(cluster=T5 {"Row"=0, "Column"=0} ("Active Cell:Active Cell"), "Row"=w996, "Column"=0 ("Row")) -> (w1001:T5)
                      n368 = Insert Into Array(array=w1006, index (row)=w996, new element=w1000) -> (w1011:string[][])  [unwired: 1 in]
                      n369 = Insert Into Array(array=w998, index=w996, new element=w996) -> (w997:i32[])
                      n370 = property on="Camera settings table" class="MCListbox (strict)"("ActiveCell"=w1001) -> ()  [unwired: 2 in, 2 out]
                    }
                    n371 = call-by-ref "?"(reference=w975, "Operation"=T6."Initialize") -> (reference out=w984:refnum<vi>, "Camera-specific out"=w973:variant)  [unwired: 14 in, 2 out]
                    n372 = Build Array (concatenate)(w993, w973) -> (w992:variant[])
                    n373 = Array Size(array=w972) -> (size(s)=w978:i32)
                    n374 = Build Array (concatenate)(w986, w984) -> (w985:refnum<vi>[])
                    n375 = Bundle By Name(cluster=cluster{"Number of channels":i32} {"Number of channels"=0}, "Number of channels"=w978) -> (w977:cluster{"Number of channels":i32})
                    n376 = Build Array (concatenate)(w981, w977) -> (w980:cluster{"Number of channels":i32}[])
                    n377 = property on="Camera settings table" class="MCListbox (strict)"("ItemNames"=w987) -> ()  [unwired: 2 in, 2 out]
                  }
                  frame True {
                  }
                }
              }
            }
          }
          frame Enabled {
          }
        }
      }
      event "16-bit mapping", "16 bit low", "16 bit high": Value Change {
        n378 = event-data() -> ()  [unwired: 1 in, 6 out]
        n379 = property on="16-bit mapping" class="Ring (strict)"() -> ("Value"=w1037:u16)  [unwired: 2 in, 2 out]
        n380 = case shown="3" w1037 {
          frame 0, Default {
            w1046 = u32 10 items=["Default"=10, "Most Significant Bits"=11, "Full Dynamic"=12, "Downshift"=13, "Given Range"=14, "90% Dynamic"=15, "Given Percent Range"=16] ("16-bit Display Mapping:Conversion Method")
            # "Full range"
            n381 = control-ref of="Image"() -> (w1047:refnum<vi>)
            n382 = property class="ImageControl"(reference=w1047, "16-bit Display Conversion Method"=w1046) -> ()  [unwired: 1 in, 2 out]
          }
          frame 1 {
            w1048 = u32 12 items=["Default"=10, "Most Significant Bits"=11, "Full Dynamic"=12, "Downshift"=13, "Given Range"=14, "90% Dynamic"=15, "Given Percent Range"=16] ("16-bit Display Mapping:Conversion Method")
            # "Full dynamic"
            n383 = control-ref of="Image"() -> (w1049:refnum<vi>)
            n384 = property class="ImageControl"(reference=w1049, "16-bit Display Conversion Method"=w1048) -> ()  [unwired: 1 in, 2 out]
          }
          frame 2 {
            w1050 = u32 15 items=["Default"=10, "Most Significant Bits"=11, "Full Dynamic"=12, "Downshift"=13, "Given Range"=14, "90% Dynamic"=15, "Given Percent Range"=16] ("16-bit Display Mapping:Conversion Method")
            # "90% dynamic"
            n385 = control-ref of="Image"() -> (w1051:refnum<vi>)
            n386 = property class="ImageControl"(reference=w1051, "16-bit Display Conversion Method"=w1050) -> ()  [unwired: 1 in, 2 out]
          }
          frame 3 {
            w1054 = u32 14 items=["Default"=10, "Most Significant Bits"=11, "Full Dynamic"=12, "Downshift"=13, "Given Range"=14, "90% Dynamic"=15, "Given Percent Range"=16] ("16-bit Display Mapping:Conversion Method")
            # "Fixed"
            n387 = control-ref of="Image"() -> (w1055:refnum<vi>)
            n388 = property on="16 bit high" class="DigNum (strict)"() -> ("Value"=w1053:i32)  [unwired: 2 in, 2 out]
            n389 = property on="16 bit low" class="DigNum (strict)"() -> ("Value"=w1052:i32)  [unwired: 2 in, 2 out]
            n390 = property class="ImageControl"(reference=w1055, "16-bit Display Conversion Method"=w1054, "16-bit Display Maximum Value"=w1053, "16-bit Display Minimum Value"=w1052) -> ()  [unwired: 1 in, 2 out]
          }
        }
      }
    }
    n391 = feedback-in #1(w119) -> ()
  }
  n392 = Destroy User Event(user event=w30) -> ()  [unwired: 1 in, 1 out]
  n393 = Destroy User Event(user event=w32) -> ()  [unwired: 1 in, 1 out]
  n394 = while "Image Processing" {
    tunnel: w10 -> [w1060]
    tunnel: [w1057] -> w9
    tunnel: w8 -> [w1057]
    tunnel: w7 -> [w1056]
    stop <- w1059 stop-if-true
    n395 = event shown="[0] Timeout" {
      selector: w1060 -> [_ _]
      dyn-events: _ -> [_ _]
      timeout: 30 -> [_ _]
      tunnel: [FALSE TRUE] -> w1059
      tunnel: w1056 -> [w1070 _]
      event Timeout {
        n396 = event-data() -> ()  [unwired: 1 in, 3 out]
        n397 = property on="Graph parameters" class="Clust (strict)"() -> ("Value"=w1064:T1)  [unwired: 2 in, 2 out]
        n398 = Unbundle By Name(w1064) -> ("Graph type"=w1063:u16, "Scale"=w1061:dbl, "Offset"=w1062:dbl)
        n399 = case shown="0, Default" w1063 {
          tunnel: w1070 -> [w1073 w1075]
          tunnel: [w1072 w1074] -> w1067
          frame 0, Default {
            n400 = call "IMAQ LinearAverages"("Image Src"=w1073) -> ("Y Axis Averages"=w1072:sgl[])  [unwired: 6 in, 4 out]
          }
          frame 1 {
            n401 = call "IMAQ LinearAverages"("Image Src"=w1075) -> ("X Axis Averages"=w1074:sgl[])  [unwired: 6 in, 4 out]
          }
        }
        n402 = Array Size(array=w1067) -> (size(s)=w1069:i32)
        n403 = for {
          N: w1069 -> [_]
          tunnel: [w1077] -> w1068 mode=indexing
          i -> [w1078]
          n404 = Increment(x=w1078) -> (x+1=w1076:i32)
          n405 = To Double Precision Float(number=w1076) -> (double precision float=w1077:dbl)
        }
        n406 = To Double Precision Float(number=w1067) -> (double precision float=w1065:dbl[])
        n407 = Build Cluster Array(w1068, w1065) -> (w1066:cluster{dbl, dbl}[])
        n408 = property on="XY Graph" class="XYGraph (strict)"("Value"=w1066, "XScale.Offset"=w1062, "XScale.Multiplier"=w1061) -> ()  [unwired: 2 in, 2 out]
      }
      event User Event {
        n409 = event-data() -> ()  [unwired: 1 in, 5 out]
      }
    }
  }
  n410 = Destroy User Event(user event=w9) -> ()  [unwired: 1 in, 1 out]
  n411 = call "IMAQ Dispose"("Image"=w50) -> ()  [unwired: 5 in, 1 out]
  n412 = flat-sequence {
    tunnel: w25 -> [w1081]
    frame #0 {
      n413 = for {
        tunnel: w1081 -> [w1083] mode=indexing
        border: 0 -> [_]
        n414 = Unbundle(w1083) -> ("Number of axes"=w1082:i32)
        n415 = for {
          N: w1082 -> [_]
          n416 = feedback #4() -> (w1084:i32)
          n417 = Increment(x=w1084) -> (x+1=w1088:i32)
          n418 = feedback-in #4(w1088) -> ()
          n419 = Bundle(w1084, 0) -> (w1086:cluster{i32, i32})  [unwired: 1 in]
          n420 = property on="Device Settings" class="MCListbox (strict)"("ActiveCell"=w1086, "CellBG"=u32 16777215) -> ()  [unwired: 2 in, 2 out]
        }
      }
    }
    frame #1 {
      n421 = property on="Device Settings" class="MCListbox (strict)"("ItemNames"=string[][] [] ("Device setup")) -> ()  [unwired: 2 in, 2 out]
    }
  }
  n422 = for {
    tunnel: w35 -> [w1094] mode=indexing
    tunnel: w34 -> [w1093] mode=indexing
    n423 = call-by-ref "?"(reference=w1094, "Device-specific in"=w1093, "Operation"=T8."Shut down") -> (reference out=w1091:refnum<vi>, error out=w1090:errorcluster)  [unwired: 6 in, 5 out]
    n424 = Close Reference(reference=w1091, error in (no error)=w1090) -> ()  [unwired: 1 out]
  }
  n425 = call-by-ref "?"(reference=w53, "Operation"=T6."Shut down", "Camera-specific in"=w48) -> (reference out=w54:refnum<vi>, error out=w55:errorcluster)  [unwired: 13 in, 2 out]
  n426 = Close Reference(reference=w54, error in (no error)=w55) -> ()  [unwired: 1 out]
